vi "FP_Tracker_v.2.2+.vi"() -> ()   [LabVIEW 2018]
uses:
  SubVi's/Controls/CTL_IO_status_indicator.ctl
  SubVi's/Controls/CTL_Zones_control_and_indicator.ctl
  SubVi's/Controls/CTL_All_References.ctl
  SubVi's/Controls/CTL_Controls_References.ctl
  SubVi's/Controls/CTL_Indicators_References.ctl
  SubVi's/Controls/CTL_Panes_and_VIs_References.ctl
  SubVi's/Controls/CTL_Cage_radial_segmentation.ctl
  SubVi's/Controls/CTL_Image_Geometrical_and_scaling_parameters.ctl
  SubVi's/Controls/CTL_Control_States.ctl
  SubVi's/Controls/CTL_States_cluster.ctl
  <vilib>/Platform/TimedLoop/XDataNode/timing_clust.ctl
  <vilib>/Platform/TimedLoop/XDataNode/nitl_modes.ctl
  <vilib>/Platform/TimedLoop/XDataNode/wakeup.ctl
  <vilib>/Utility/error.llb/DialogType.ctl
  SubVi's/Controls/CTL_Acquisition_speed_selector.ctl
  <vilib>/Instr/_visa.llb/VISA Flush IO Buffer Mask.ctl
  <extravilib>/ChannelInstances/Lossy Stream-c(dbl,dbl,sgl,dbl,dbl,dbl,sgl,dbl)/Read With Abort.vi
  <extravilib>/ChannelInstances/Lossy Stream-c(dbl,dbl,sgl,dbl,dbl,dbl,sgl,dbl)/Write With Abort.vi
  <extravilib>/ChannelInstances/Lossy Stream-c(dbl,dbl,sgl,dbl,dbl,dbl,sgl,dbl)/EndpointRead.vi
  <extravilib>/ChannelInstances/Lossy Stream-c(dbl,dbl,sgl,dbl,dbl,dbl,sgl,dbl)/Endpoint.vi
  <extravilib>/ChannelInstances/Lossy Stream-c(dbl,dbl,sgl,dbl,dbl,dbl,sgl,dbl)/Instantiate.vi
  SubVi's/SW_Globals_2.2+.vi
  <vilib>/Platform/TimedLoop/scheduler/LVUserAPI/_suppVIs/Create_1kHz_TSource.vi
  <extravilib>/ChannelInstances/Lossy Stream-c(dbl,dbl,sgl,dbl,dbl,dbl,sgl,dbl)/)Channel.vi
  <resource>/ChannelSupport/_ChannelSupport/WaitIfNeeded.vi
  <vilib>/nisyscfg/Close (Resources).vi
  <vilib>/nisyscfg/Close (System).vi
  <vilib>/platform/TimedLoop/XDataNode/XDataNode.xnode
  <vilib>/Platform/TimedLoop/XDataNode/XDNodeRunTimeDep.lvlib
  <extravilib>/ChannelInstances/Lossy Stream-c(dbl,dbl,sgl,dbl,dbl,dbl,sgl,dbl).lvlib
  <vilib>/nisyscfg/nisyscfg.lvlib
  <resource>/objmgr/nisysapi.rc
  <resource>/objmgr/nicontrollersysapi.rc
  <vilib>/Utility/config.llb/NI_LVConfig.lvlib
panel:
  out "CPU load":sgl(slide) scale=0.0..100.0
  in  "ROIs list":i32(listbox)
  out "ROIs":T1
  out "Rainbow track (l.v.o.)":bool=TRUE
  out "Colors array (l.v.o.)":u32[](array[colorbox])
  out "UI update period (l.v.o.)":i64=53
  out "Trace length, samples (l.v.o)":u16(slide)=20 scale=0.0..2000.0
  out "Bright mouse lineout (l.v.o.)":bool
  out "Img geom and scaling (l.v.o.)":T2
  out "SG coeff. 0th order (l.v.o.)":dbl[](array[numeric])
  out "Ports IO config (l.v.o.)":bool[](array[boolean])
  out "SB size (l.v.o.)":u8
  out "VISA resource name":refnum<visa-resource-name>
  out "Cage size":string="Large" caption="Cage diameter"
  in  "Set/Rec and Analyse Tab":enum32{"Settings", "Recording and Analysis"}(tab)
  in  "Set IO config":bool
  in  "Save settings":bool
  in  "Reset zones":bool
  out "Ready":bool=TRUE
  in  "Check HW connection":bool
  in  "Reset stimuli":bool
  in  "Cage radial segmentation":T3={"CENTER"={"Radius, mm CENTER"=30}, "MIDFIELD"={"Radius, mm MIDFIELD"=75, "N segments MIDFIELD"=2, "Starting angle MIDFIELD"=0}, "BORDER"={"N segments BORDER"=4, "Starting angle BORDER"=0}} caption="Radial segmentation" {"BORDER"."N segments BORDER" min=1 max=12; "MIDFIELD"."N segments MIDFIELD" max=8; "CENTER"."Radius, mm CENTER" min=5 step=1}
  in  "Stimulus presets (RZ)":T4(array[cluster]) {"TTL out" items=["1"=1, "2"=2, "1 + 2"=3]; "Stimulus, s" min=0 max=10000 step=0.1; "Time, s" min=0 max=10000 step=0.1; "Event type" items=["Time spent in zone", "Future options"]}
  in  "Rainbow track":bool caption="Rainbow"
  in  "Show magnets":bool=TRUE caption="Magnets"
  in  "Playback speed":u16(ring)=3 caption="Speed" items=["25"=75, "10"=30, "6"=18, "4"=12, "2"=6, "1"=3, "2/3"=2, "1/3"=1]
  in  "Show heatmap":bool caption="Heat map"
  in  "Show full track":bool caption="Full track"
  in  "Show zones":bool=TRUE caption="Zones"
  in  "Trace, s":u16(slide)=5 max=30 step=1 scale=0.0..30.0
  out "Mouse speed, mm/s":dbl=0.28949046360238656 caption="Mouse speed" format="%05.1f"
  in  "Multiplyer of chart RX":u8(slide)=1 min=1 max=10 step=1 scale=1.0..6.0
  out "Running, perc. of time":dbl=0.28949046360238656 caption="Run, %" format="%05.2f"
  out "Mouse speed":waveform(dbl)(graph)={"t0"=timestamp(3610093053.229 s since 1904-01-01), "dt"=1.0, "Y"=[0.28949046360238656]}
  out "Histograms":dbl[](graph) caption="Zone preference (normalized)"
  in  "Reset barplot":bool
  out "Timing Source":string
  in  "Panes references":T5
  in  "Indicators references":T6
  in  "Controls references":T7
  in  "All references":T8
  in  "Experiment Diagram":T9(plugin-control)=refnum
  out "HW info":string
  out "Port":string="Large"
  in  "Timeline":dbl(slide) min=0.0 step=1.0 scale=0.0..3599.0 scale format="%<%H:%M:%S>t"
  in  "Play/Pause":bool
  in  "Open File":bool
  out "Record timestamp":dbl format="%<%H:%M:%S%3u>t"
  out "Current Time":timestamp=timestamp(3610093053.229 s since 1904-01-01) format="%<%H:%M:%S %d.%m.%Y>T"
  out "Current zone":T10={"01"=TRUE, "02"=TRUE, "03"=TRUE, "04"=TRUE, "05"=TRUE, "06"=TRUE, "07"=TRUE, "08"=TRUE, "09"=TRUE, "10"=TRUE, "11"=TRUE, "12"=TRUE, "13"=TRUE}
  in  "Record/Stop":bool
  in  "By Zone stim. setup":T11=enum."Zone 13"
  out "IO status indicator":T12
  in  "error in (no error)":errorcluster
  out "error out":errorcluster={"status"=TRUE, "code"=1, "source"="Dequeue Element in NI_LVConfig.lvlib:Read Value Without Comment.vi->NI_LVConfig.lvlib:Read Key (I32).vi->SW_Load_settings_to_main_tab.vi"}
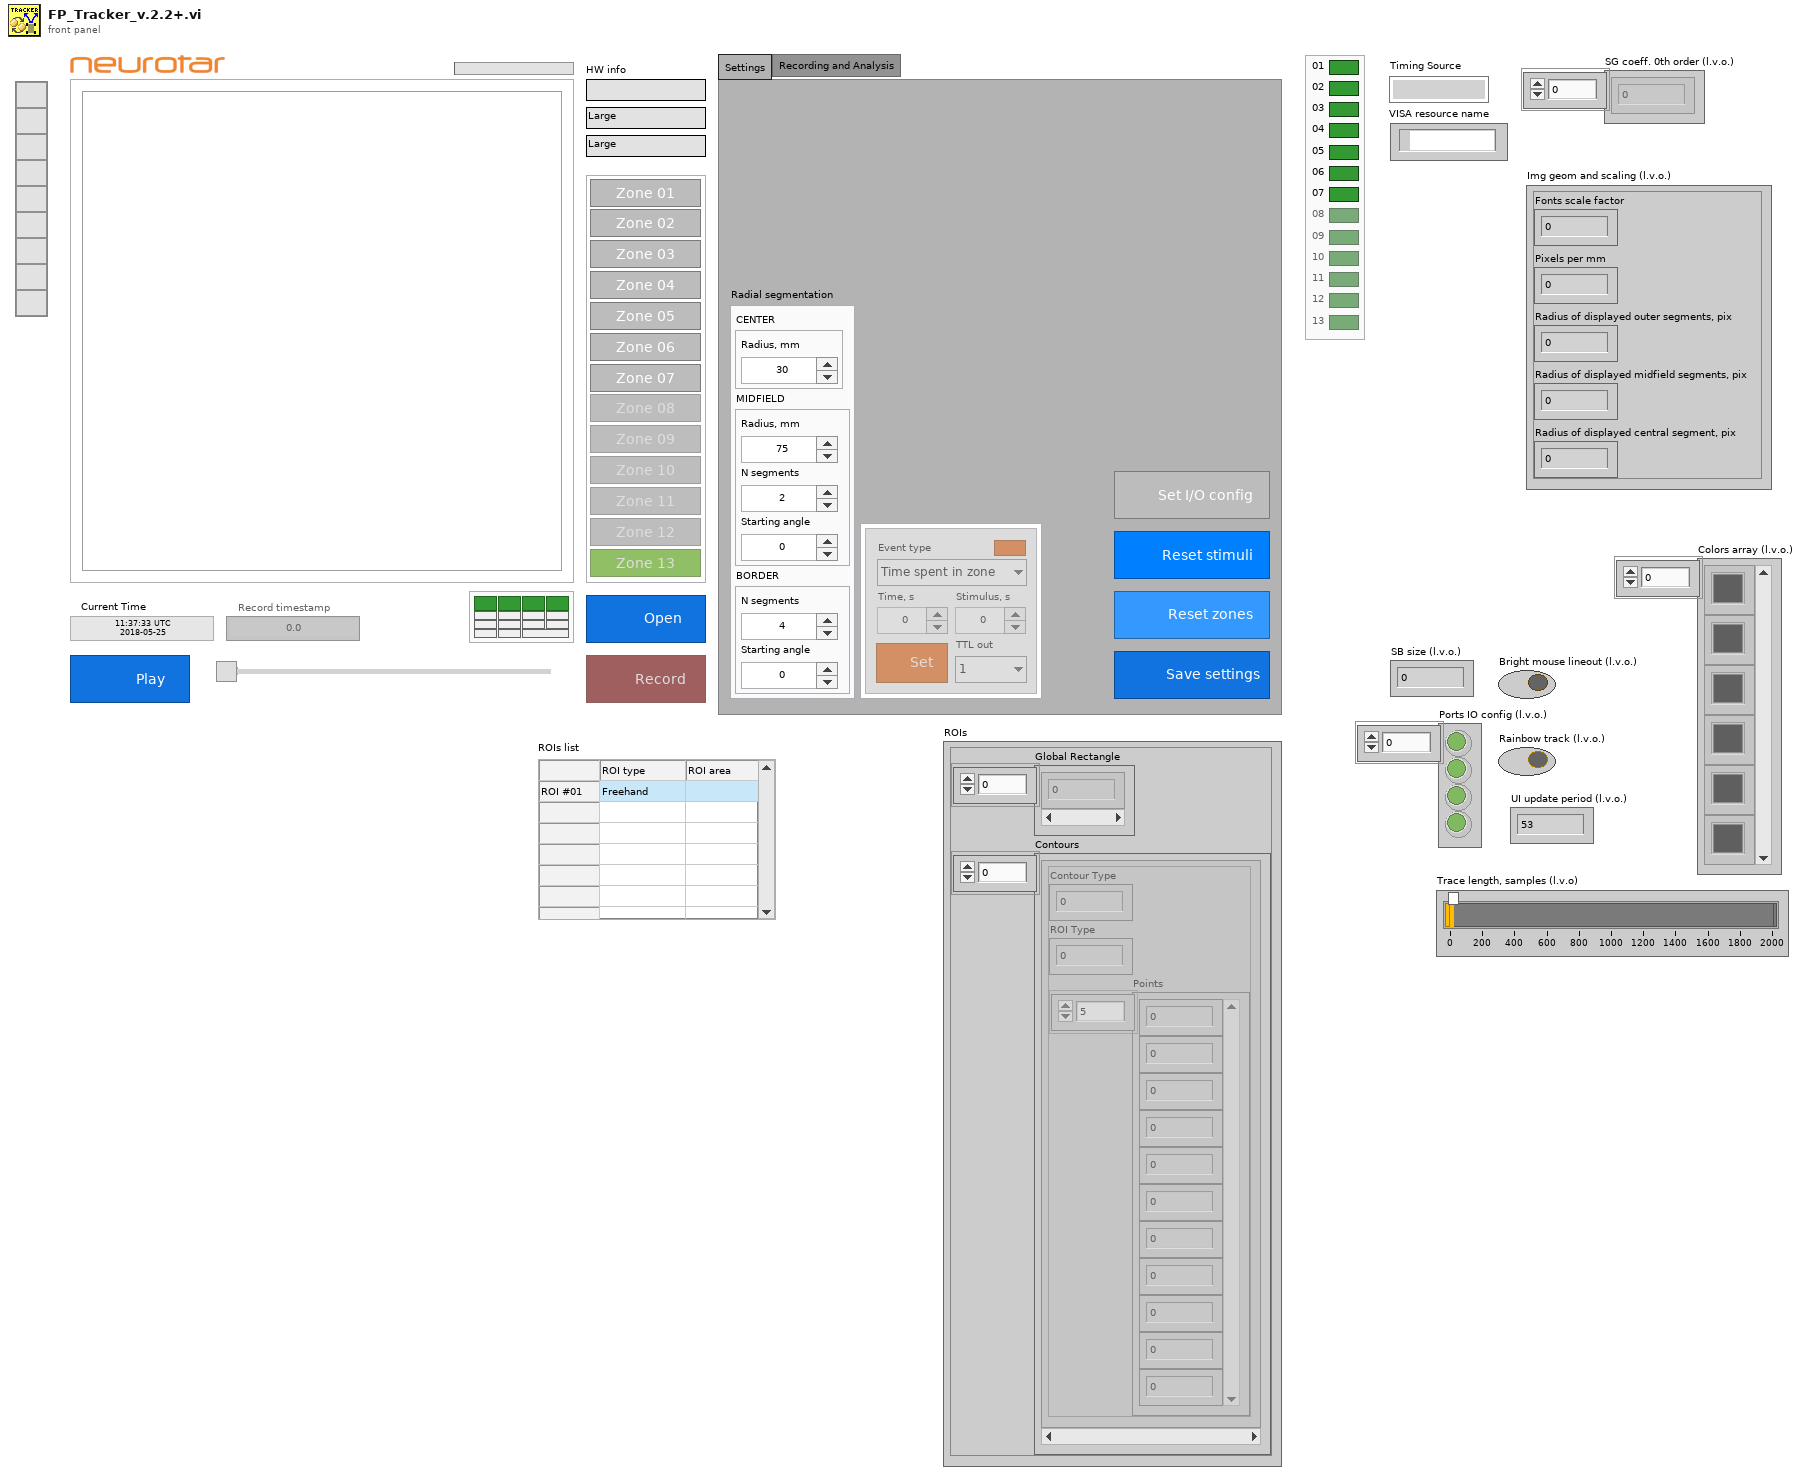
[diagram p1: front panel]
types:
  T1 = cluster{"Global Rectangle":i32[], "Contours":cluster{"Contour Type":u32, "ROI Type":u32, "Points":i32[]}[]}
  T2 = typedef "CTL_Image_Geometrical_and_scaling_parameters.ctl" = cluster{"Fonts scale factor":dbl, "Pixels per mm":dbl, "Radius of displayed outer segments, pix":dbl, "Radius of displayed midfield segments, pix":dbl, "Radius of displayed central segment, pix":dbl}
  T3 = typedef "CTL_Cage_radial_segmentation.ctl" = cluster{"CENTER":cluster{"Radius, mm CENTER":u16}, "MIDFIELD":cluster{"Radius, mm MIDFIELD":u16, "N segments MIDFIELD":u8, "Starting angle MIDFIELD":i16}, "BORDER":cluster{"N segments BORDER":u8, "Starting angle BORDER":i16}}
  T4 = cluster{"Event type":u16, "Time, s":sgl, "Stimulus, s":sgl, "Set/Clear":bool, "TTL out":u16, "Stim. has been set":bool}[]
  T5 = typedef "CTL_Panes_and_VIs_References.ctl" = cluster{"Pane":refnum<vi>, "This VI":refnum<vi>, "Menu":refnum<k9>}
  T6 = typedef "CTL_Indicators_References.ctl" = cluster{"HW info":refnum<vi>, "Port":refnum<vi>, "Ready":refnum<vi>, "IO status indicator":refnum<vi>, "Current Time":refnum<vi>, "Record timestamp":refnum<vi>, "Mouse speed":refnum<vi>, "Mouse speed, mm/s":refnum<vi>, "Running, perc. of time":refnum<vi>, "Histograms":refnum<vi>, "Cage size":refnum<vi>}
  T7 = typedef "CTL_Controls_References.ctl" = cluster{"Check HW connection":refnum<vi>, "Start Tracking button":refnum<vi>, "Reset zones":refnum<vi>, "Reset stimuli":refnum<vi>, "Record/Stop":refnum<vi>, "Reset barplot":refnum<vi>, "Multiplyer of chart RX":refnum<vi>, "Show zones":refnum<vi>, "Show magnets":refnum<vi>, "Show heatmap":refnum<vi>, "Show full track":refnum<vi>, "Open File":refnum<vi>, "Play/Pause":refnum<vi>, "Trace, s":refnum<vi>, "Playback speed":refnum<vi>, "Timeline":refnum<vi>, "By Zone stim. setup":refnum<vi>, "Set, Rec and Analyse Tab":refnum<vi>, "Cage radial segmentation":refnum<vi>, "Set IO config":refnum<vi>, "Rainbow track":refnum<vi>}
  T8 = typedef "CTL_All_References.ctl" = cluster{"Controls references":T7, "Indicators references":T6, "Service references":T5}
  T9 = typedef "IMAQ Image.ctl" = refnum<image>
  T10 = cluster{"01":bool, "02":bool, "03":bool, "04":bool, "05":bool, "06":bool, "07":bool, "08":bool, "09":bool, "10":bool, "11":bool, "12":bool, "13":bool}
  T11 = typedef "CTL_Zones_control_and_indicator.ctl" = enum32{"No Selection", "Zone 01", "Zone 02", "Zone 03", "Zone 04", "Zone 05", "Zone 06", "Zone 07", "Zone 08", "Zone 09", "Zone 10", "Zone 11", "Zone 12", "Zone 13"}
  T12 = typedef "CTL_IO_status_indicator.ctl" = cluster{"IO1":bool, "IO2":bool, "IO3":bool, "IO4":bool, "St1":bool, "St2":bool, "St3":bool, "St4":bool, "Z1":bool, "Z2":bool, "Z3":bool, "Z4":bool, "Syn1":bool, "Syn2":bool, "RS-232 ext. activated":bool}
  T13 = cluster{"HW info":refnum<vi>, "Port":refnum<vi>, "Ready":refnum<vi>, "IO status indicator":refnum<vi>, "Current Time":refnum<vi>, "Record timestamp":refnum<vi>, "Mouse speed":refnum<vi>, "Mouse speed, mm/s":refnum<vi>, "Running, perc. of time":refnum<vi>, "Histograms":refnum<vi>, "Cage size":refnum<vi>}
  T14 = cluster{"Pane":refnum<vi>, "This VI":refnum<vi>, "menu reference":refnum<k9>}
  T15 = cluster{"Check HW connection":refnum<vi>, "Save settings":refnum<vi>, "Reset zones":refnum<vi>, "Reset stimuli":refnum<vi>, "Record/Stop":refnum<vi>, "Reset barplot":refnum<vi>, "Multiplyer of chart RX":refnum<vi>, "Show zones":refnum<vi>, "Show magnets":refnum<vi>, "Show heatmap":refnum<vi>, "Show full track":refnum<vi>, "Open File":refnum<vi>, "Play/Pause":refnum<vi>, "Trace, s":refnum<vi>, "Playback speed":refnum<vi>, "Timeline":refnum<vi>, "By Zone stim. setup":refnum<vi>, "Set/Rec and Analyse Tab":refnum<vi>, "Cage radial segmentation":refnum<vi>, "Set IO config":refnum<vi>, "Rainbow track":refnum<vi>}
  T16 = typedef "CTL_States_cluster.ctl" = cluster{"Acq. is ON":bool, "Playing loaded":bool, "Recording now":bool, "Has been recorded":bool, "Data saved":bool, "Data loaded":bool, "Stop and Exit":bool}
  T17 = typedef "CTL_Control_States.ctl" = enum16{"SW Init", "HW Init", "Close App", "Update port info (Init OK)", "Unlock UI (init OK)", "Save HW Settings", "Re-check HW (init failed)", "Configure port(s)", "Zones layout update", "Set I/O config", "Reset stimulus", "Reset zones", "Play Start", "Play Stop", "Upd. trace length", "Cage and recording settings", "Update filter"}
  T18 = typedef "XDNodeRunTimeDep.lvlib/timing_clust.ctl" = cluster{"Expected End [f-1]":u64, "Actual End [f-1]":u64, "Finished Late? [f-1]":bool, "Expected End [i-1]":u64, "Actual End [i-1]":u64, "Finished Late? [i-1]":bool, "Expected Start [i]":u64, "Actual Start [i]":u64, "Expected Start [f]":u64, "Actual Start [f]":u64, "Source Name":string, "Structure Name":string, "Period":i64, "Deadline":i64, "Offset":i64, "Start":i64, "Priority":i32, "Timeout":i32, "Mode":T19, "Wakeup Reason":T20, "Error":errorcluster, "Source Type":string, "Secondary Source Type":string, "Global End Time":u64, "Global Start Time":u64, "Frame Duration":u64, "Iteration Duration":u64, "Assigned CPU":i32, "I/O Scan Engine Mode":u32}
  T19 = typedef "XDNodeRunTimeDep.lvlib/nitl_modes.ctl" = enum32{"No Change", "Process missed periods, maintain original phase", "Discard missed periods, maintain original phase", "Process missed periods, ignore original phase", "Discard missed periods, ignore original phase"}
  T20 = typedef "XDNodeRunTimeDep.lvlib/wakeup.ctl" = enum32{"Normal", "Aborted", "Asynchronous wakeup", "Timing source error", "Timed loop error", "Timeout"}
  T21 = cluster{"Contour Type":u32, "ROI Type":u32, "Points":i32[]}[]
  T22 = typedef "CTL_Settings_cluster.ctl" = cluster{"Defaults":cluster{"Default User":dbl, "VISA Resource Name ":string}, "Recording and saving":cluster{"Researcher name":string, "Name prefix":string, "Data filtering":T23, "Stop at":dbl, "\"Stop at\" enabled":bool, "Default save folder path":path}, "Geometry":T24, "IO parameters":T25, "Stimulus presets array":T26[], "Settings loaded OK":bool}
  T23 = typedef "CTL_Filter_selector.ctl" = cluster{"Filter type":enum16{"None", "Savitzky-Golay"}, "Length":i32, "Order":i32}
  T24 = typedef "CTL_Segmented_plot_parameters.ctl" = cluster{"Cage diameter, mm":u16, "Starting angle MIDFIELD":i16, "Starting angle BORDER":i16, "Radius, mm CENTER":u16, "Radius, mm MIDFIELD":u16, "N segments MIDFIELD":u8, "N segments BORDER":u8, "R-gap, mm":sgl, "Bridge swap":bool, "Bridge H. offset":sgl, "Bridge V. offset":sgl, "Twisted neck":bool, "Alt. magn. orientation":bool}
  T25 = typedef "CTL_IO_params_cluster.ctl" = cluster{"IO general config.":u16, "IO 1 configuration":u16, "IO 2 configuration":u16, "IO 3 configuration":u16, "IO 4 configuration":u16, "Activate ext. RS-232":u16, "IO inversion config.":u16, "Sync capability":u8}
  T26 = typedef "CTL_Single_stimulus_setting.ctl" = cluster{"Event type":u16, "Dur., s":sgl, "Stim., s":sgl, "TTL out N":u16, "Set/Clear":bool, "Stim. has been set":bool}
  T27 = cluster{"Radius, mm MIDFIELD":u16, "N segments MIDFIELD":u8, "Starting angle MIDFIELD":i16}
  T28 = cluster{"N segments BORDER":u8, "Starting angle BORDER":i16}
  T29 = cluster{"Numeric Control":u32, "Numeric Control":u32}[]
  T30 = typedef "CTL_Acquisition_speed_selector.ctl" = enum16{"Max", "High stability", "Eco"}
  T31 = enum32{"Page Enabled", "Page Disabled", "Page Disabled & Grayed"}
  T32 = enum8{"Enabled", "Disabled", "Disabled and Grayed Out"}
  T33 = typedef "DialogType.ctl" = u16
  T34 = enum32{"invalid app kind", "Development System", "Run Time System", "Student Edition", "Embedded LabVIEW", "Evaluation", "Custom"}
  T35 = typedef "CTL_Paths_cluster.ctl" = cluster{"Temporary file output path":path, "Density map array output path":path, "Recording settings output path":path, "Density map picture output path":path, "Layout picture output path":path, "Path to the settings file":path, "Path to TDMS file":path, "TDMS file reference":refnum<k34>, "Default save folder path":path}
  T36 = cluster{"Default User":dbl, "VISA Resource Name ":string}
  T37 = typedef "NI_LVConfig.lvlib/Config Data RefNum.ctl" = refnum<k1>
  T38 = typedef "VISA Flush IO Buffer Mask.ctl" = u16
  T39 = cluster{"ms since ON":u32, "delta time":u32, "X1":sgl, "Y1":sgl, "X2":sgl, "Y2":sgl, "TTL inputs":u8, "TTL outputs":u8, "Frame timestamp":timestamp, "Frame OK":bool}
  T40 = cluster{"ms since ON":u32, "delta time":u32, "X1":sgl, "Y1":sgl, "X2":sgl, "Y2":sgl, "TTL in 1":i16, "TTL in 2":i16, "Frame timestamp":timestamp, "Frame OK":bool}
  T41 = cluster{"R from center":dbl, "sin(a)":dbl, "Mouse Xc":dbl, "Mouse Yc":dbl, "X1-X2":dbl, "Y1-Y2":dbl, "Cage Xc":dbl, "Cage Yc":dbl}
  T42 = cluster{"R from center":dbl, "phi (mouse angular position in the cage)":dbl, "alpha (mouse rot. angle)":sgl, "X":dbl, "Y":dbl, "theta (from center towards mouse)":dbl, "beta (cage rot. against mouse)":sgl, "w (mouse angle to wall)":dbl}
  T43 = typedef "Lossy Stream-c(dbl,dbl,sgl,dbl,dbl,dbl,sgl,dbl).lvlib/)Channel.ctl" = refnum<queue>
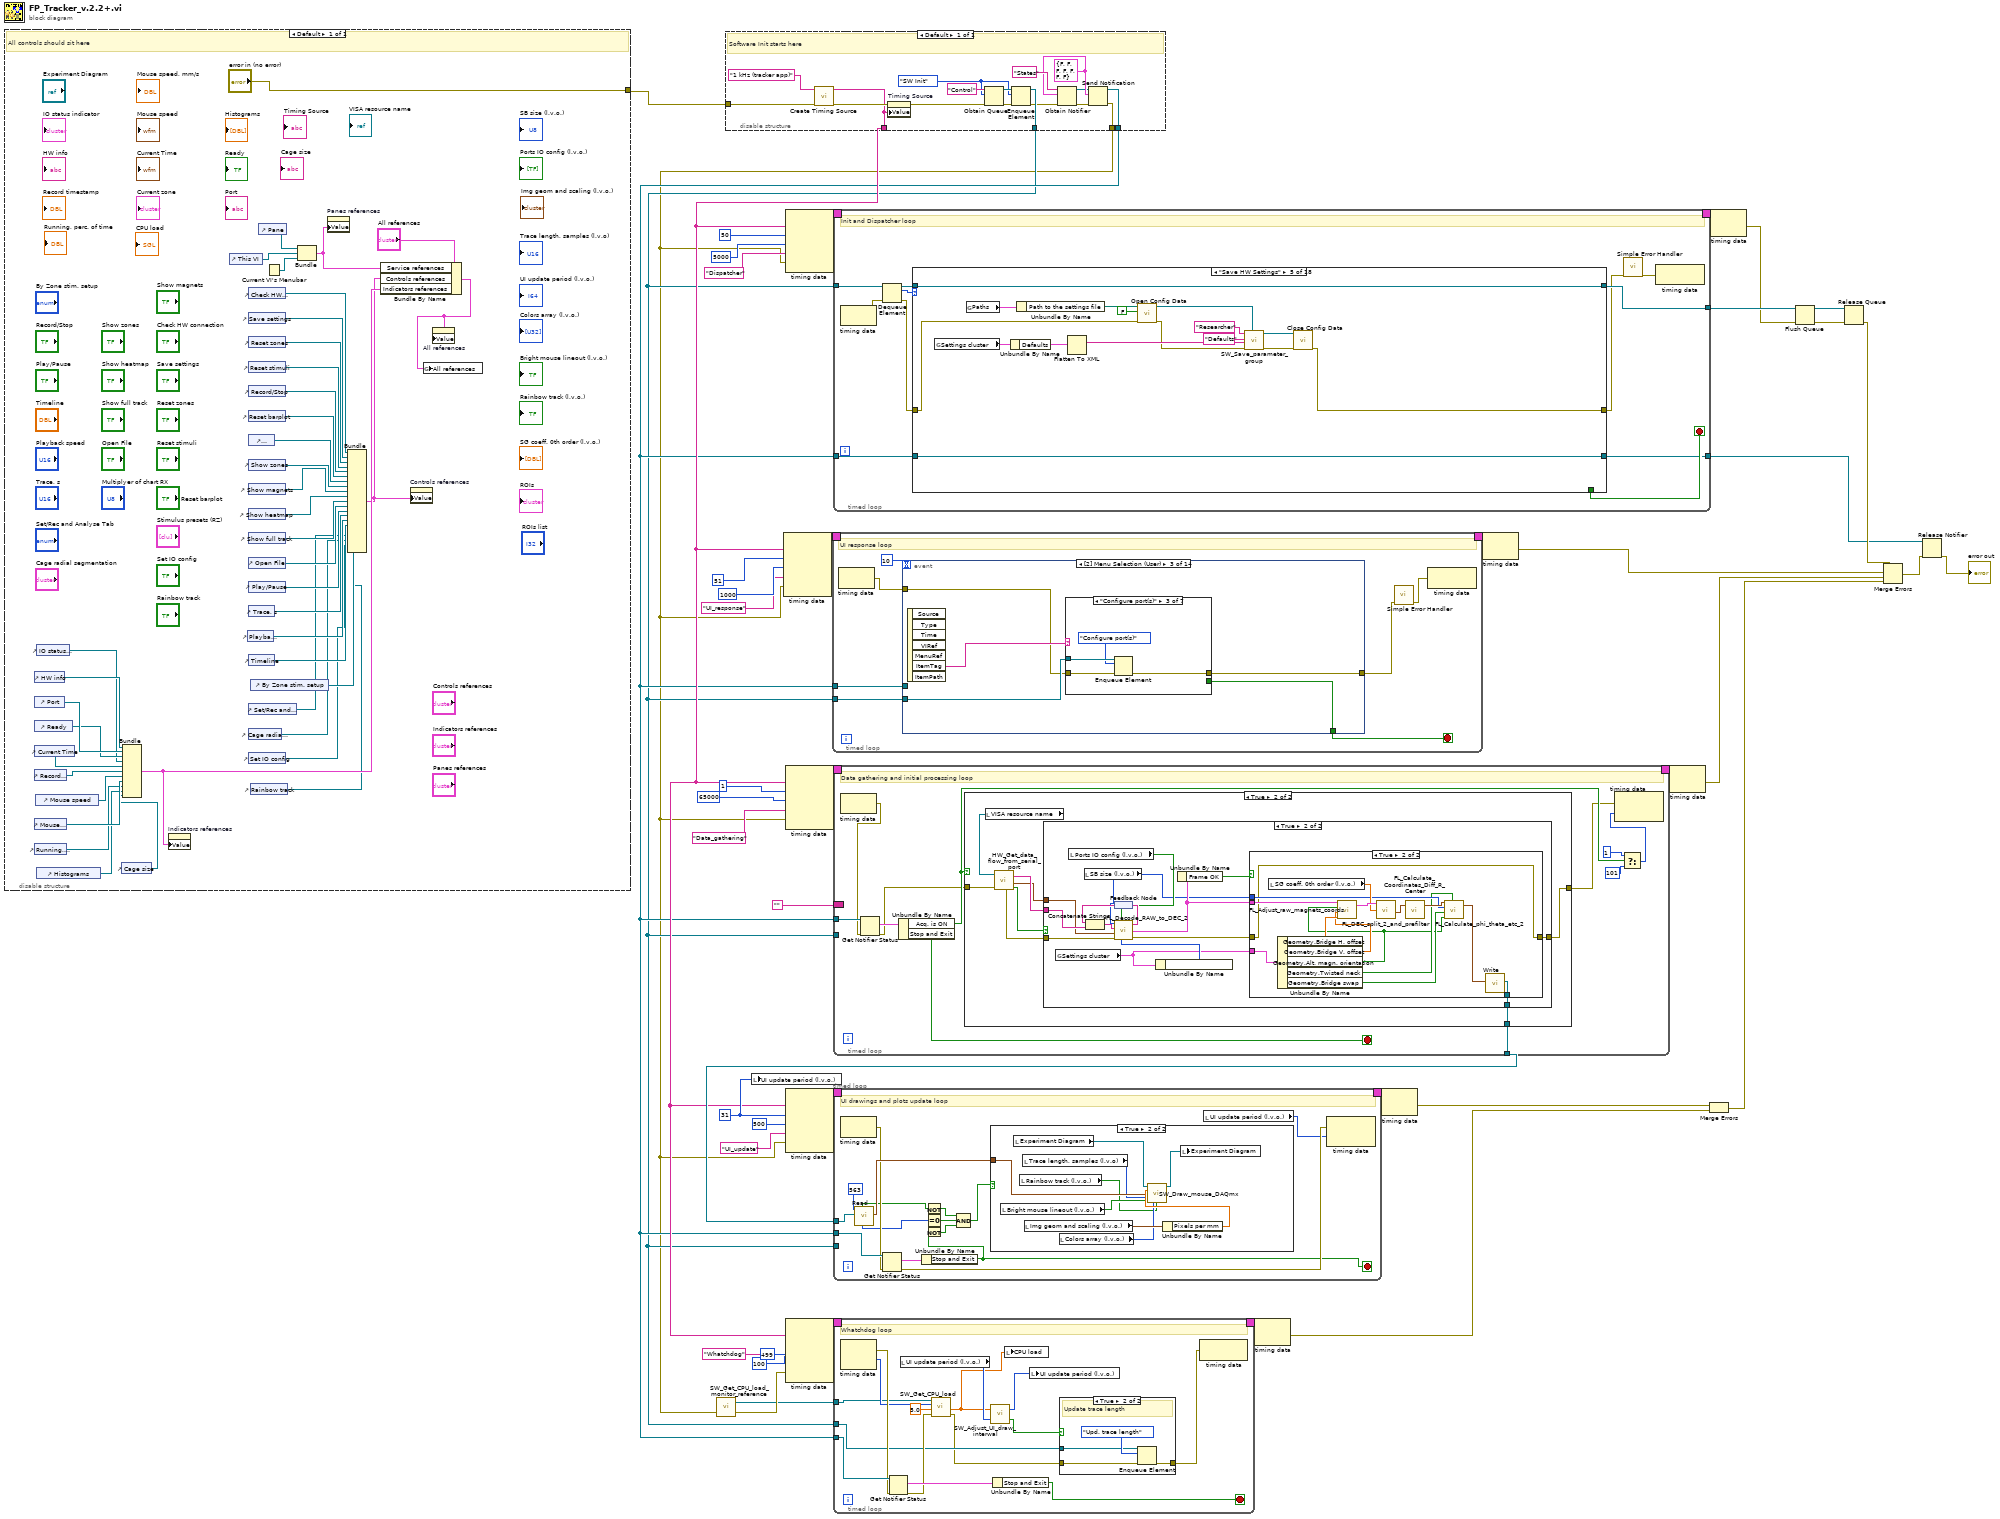
[diagram p0: block diagram]
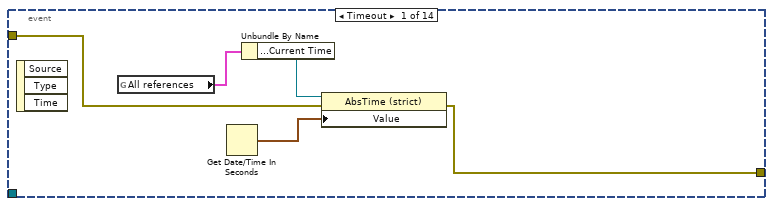
[diagram p7: hidden frame]
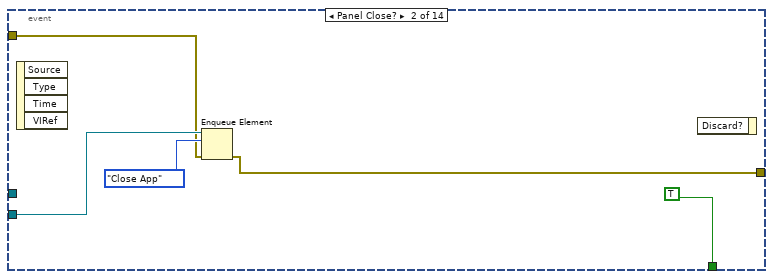
[diagram p8: hidden frame]
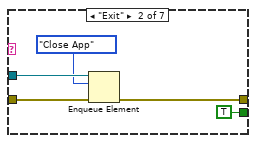
[diagram p10: hidden frame]
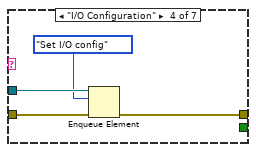
[diagram p11: hidden frame]
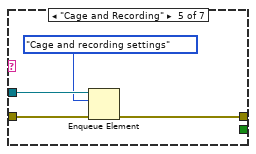
[diagram p12: hidden frame]
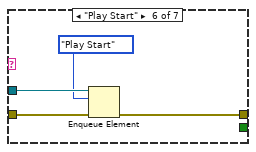
[diagram p13: hidden frame]
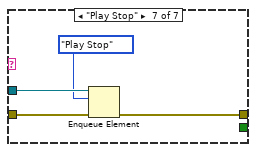
[diagram p14: hidden frame]
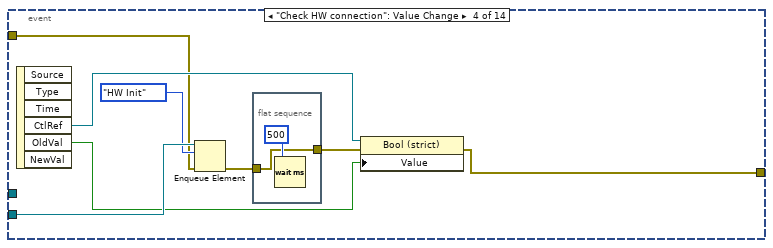
[diagram p15: hidden frame]
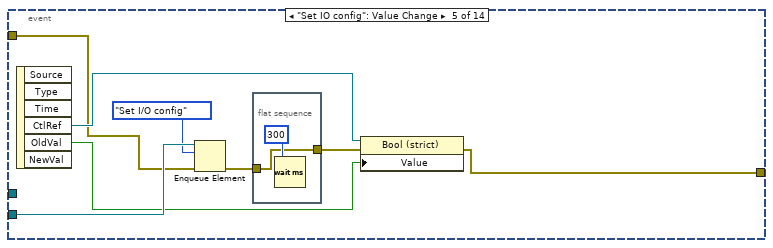
[diagram p16: hidden frame]
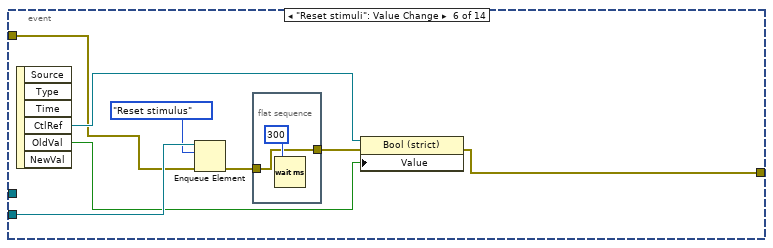
[diagram p17: hidden frame]
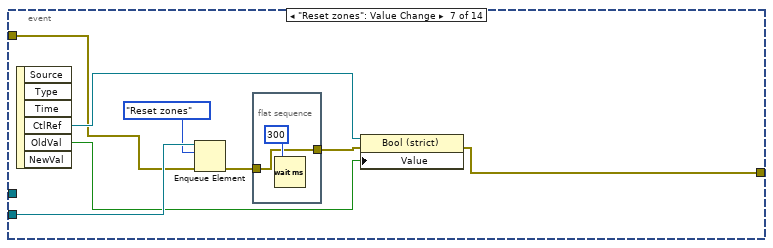
[diagram p18: hidden frame]
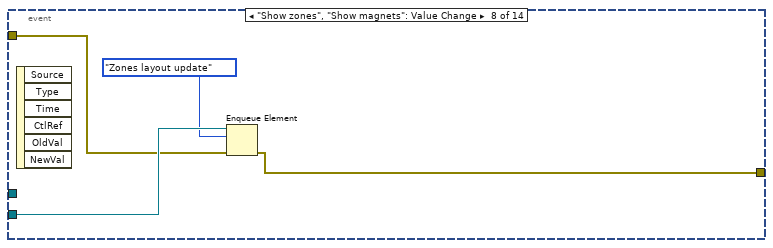
[diagram p19: hidden frame]
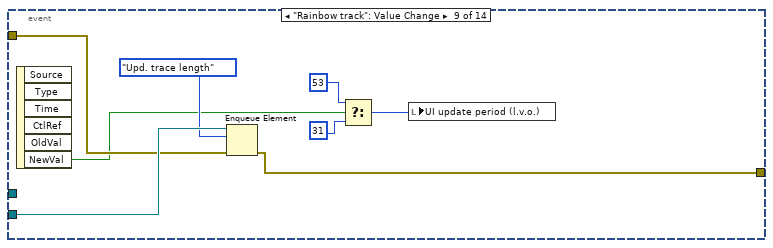
[diagram p20: hidden frame]
diagram:
  w23 = i64 31 ("Period")
  n1 = disable-structure shown="Default" {
    disable-tunnel: ["error in (no error)"] -> w29
    frame Enabled {
      # "All controls should sit here"
      n2 = control-ref of="Record timestamp"() -> (w67:refnum<vi>)
      n3 = control-ref of="Mouse speed, mm/s"() -> (w65:refnum<vi>)
      n4 = control-ref of="Running, perc. of time"() -> (w64:refnum<vi>)
      n5 = control-ref of="HW info"() -> (w71:refnum<vi>)
      n6 = control-ref of="Port"() -> (w70:refnum<vi>)
      n7 = control-ref of="Ready"() -> (w69:refnum<vi>)
      n8 = control-ref of="Current Time"() -> (w68:refnum<vi>)
      n9 = control-ref of="Mouse speed"() -> (w66:refnum<vi>)
      n10 = control-ref of="IO status indicator"() -> (w59:refnum<vi>)
      n11 = control-ref of="Histograms"() -> (w63:refnum<vi>)
      n12 = control-ref of="Cage size"() -> (w50:refnum<vi>)
      n13 = Bundle("HW info"=w71, "Port"=w70, "Ready"=w69, "IO status indicator"=w59, "Current Time"=w68, "Record timestamp"=w67, "Mouse speed"=w66, "Mouse speed, mm/s"=w65, "Running, perc. of time"=w64, "Histograms"=w63, "Cage size"=w50) -> (w56:T13)  [unwired: 1 in]
      n14 = property on="Indicators references" class="Clust (strict)"("Value"=w56) -> ()  [unwired: 2 in, 2 out]
      n15 = control-ref of="This VI"() -> (w61:refnum<vi>)
      n16 = control-ref of="Playback speed"() -> (w74:refnum<vi>)
      n17 = control-ref of="Check HW connection"() -> (w87:refnum<vi>)
      n18 = control-ref of="Save settings"() -> (w86:refnum<vi>)
      n19 = control-ref of="Reset zones"() -> (w85:refnum<vi>)
      n20 = control-ref of="Reset stimuli"() -> (w84:refnum<vi>)
      n21 = control-ref of="Record/Stop"() -> (w83:refnum<vi>)
      n22 = control-ref of="Reset barplot"() -> (w82:refnum<vi>)
      n23 = control-ref of="Multiplyer of chart RX"() -> (w81:refnum<vi>)
      n24 = control-ref of="Show zones"() -> (w80:refnum<vi>)
      n25 = control-ref of="Show magnets"() -> (w60:refnum<vi>)
      n26 = control-ref of="Show heatmap"() -> (w79:refnum<vi>)
      n27 = control-ref of="Show full track"() -> (w78:refnum<vi>)
      n28 = control-ref of="Open File"() -> (w77:refnum<vi>)
      n29 = control-ref of="Play/Pause"() -> (w76:refnum<vi>)
      n30 = control-ref of="Trace, s"() -> (w75:refnum<vi>)
      n31 = control-ref of="Timeline"() -> (w73:refnum<vi>)
      n32 = control-ref of="Set/Rec and Analyse Tab"() -> (w54:refnum<vi>)
      n33 = control-ref of="Cage radial segmentation"() -> (w53:refnum<vi>)
      n34 = control-ref of="Set IO config"() -> (w52:refnum<vi>)
      n35 = control-ref of="By Zone stim. setup"() -> (w72:refnum<vi>)
      n36 = control-ref of="Rainbow track"() -> (w48:refnum<vi>)
      n37 = control-ref of="Pane"() -> (w62:refnum<vi>)
      n38 = Current VI's Menubar() -> (w49:refnum<k9>)
      n39 = Bundle("Pane"=w62, "This VI"=w61, "menu reference"=w49) -> (w57:T14)  [unwired: 1 in]
      n40 = property on="Panes references" class="Clust (strict)"("Value"=w57) -> ()  [unwired: 2 in, 2 out]
      n41 = Bundle("Check HW connection"=w87, "Save settings"=w86, "Reset zones"=w85, "Reset stimuli"=w84, "Record/Stop"=w83, "Reset barplot"=w82, "Multiplyer of chart RX"=w81, "Show zones"=w80, "Show magnets"=w60, "Show heatmap"=w79, "Show full track"=w78, "Open File"=w77, "Play/Pause"=w76, "Trace, s"=w75, "Playback speed"=w74, "Timeline"=w73, "By Zone stim. setup"=w72, "Set/Rec and Analyse Tab"=w54, "Cage radial segmentation"=w53, "Set IO config"=w52, "Rainbow track"=w48) -> (w51:T15)  [unwired: 1 in]
      n42 = Bundle By Name(cluster="All references", "Service references"=w57, "Controls references"=w51, "Indicators references"=w56) -> (w55:T8)
      n43 = property on="Controls references" class="Clust (strict)"("Value"=w51) -> ()  [unwired: 2 in, 2 out]
      n44 = global write "SW_Globals_2.2+.vi" "All references"(w55) -> ()
      n45 = property on="All references" class="Clust (strict)"("Value"=w55) -> ()  [unwired: 2 in, 2 out]
    }
  }
  n46 = disable-structure shown="Default" {
    disable-tunnel: w29 -> [w98]
    disable-tunnel: [w97] -> w6
    disable-tunnel: [w96] -> w11
    disable-tunnel: [w90] -> w7
    disable-tunnel: [w89] -> w3
    frame Enabled {
      w92 = T16 {"Acq. is ON"=FALSE, "Playing loaded"=FALSE, "Recording now"=FALSE, "Has been recorded"=FALSE, "Data saved"=FALSE, "Data loaded"=FALSE, "Stop and Exit"=FALSE} ("States cluster")
      w99 = CTL_Control_States."SW Init"
      # "Software Init starts here"
      n47 = call-poly <vilib>:"Create Timing Source.vi"("error in (no error)"=w98, "name (in)"="1 kHz (tracker app)") -> ("error out"=w105:errorcluster, "name (out)"=w96:string)  [unwired: 8 in]
      n48 = property on="Timing Source" class="Str"(error in=w105, "Value"=w96) -> (error out=w103:errorcluster)  [unwired: 1 in, 1 out]
      n49 = Obtain Queue(name (unnamed)="Control", element data type=w99, error in (no error)=w103) -> (queue out=w100:refnum<queue>, error out=w101:errorcluster)  [unwired: 2 in, 1 out]
      n50 = Enqueue Element(queue=w100, element=w99, error in (no error)=w101) -> (queue out=w97:refnum<queue>, error out=w95:errorcluster)  [unwired: 1 in, 1 out]
      n51 = Obtain Notifier(name (unnamed)="States", notification data type=w92, error in (no error)=w95) -> (notifier out=w91:refnum<notifier>, error out=w93:errorcluster)  [unwired: 1 in, 1 out]
      n52 = Send Notification(notification=w92, notifier=w91, error in (no error)=w93) -> (notifier out=w90:refnum<notifier>, error out=w89:errorcluster)
    }
  }
  n53 = call "SW_Get_CPU_load_monitor_reference.vi"("error in (no error)"=w3) -> ("error out"=w2:errorcluster, "CPU monitor .NET reference"=w1:refnum<k24>)  [unwired: 1 in]
  n54 = local write "UI update period (l.v.o.)"(w23) -> ()
  n55 = node-c288(w11, i64 51 ("Period"), 1000 ("Priority"), "UI_response" ("Structure Name"), w3) -> (w40:T18)
  n56 = node-c288(w11, i64 50 ("Period"), 5000 ("Priority"), "Dispatcher" ("Structure Name"), w3) -> (w47:T18)
  n57 = node-c288(w11, i64 1 ("Period"), 65000 ("Priority"), "Data_gathering" ("Structure Name"), w3) -> (w35:T18)
  n58 = node-c288(w11, w23, 500 ("Priority"), "UI_update" ("Structure Name"), w3) -> (w28:T18)
  n59 = node-c288(w11, i64 499 ("Period"), 100 ("Priority"), "Whatchdog" ("Structure Name"), w2) -> (w13:T18)
  n60 = timed-loop {
    timing: w40 -> [_]
    timing-out: [_] -> w39
    tunnel: w6 -> [w111]
    tunnel: w7 -> [w109]
    stop <- w112 stop-if-true
    # "UI response loop"
    n61 = node-c288() -> (w107:errorcluster)  [unwired: 1 in]
    n62 = event shown="[2] Menu Selection (User)" {
      selector: _ -> [_ _ _ _ _ _ _ _ _ _ _ _ _ _]
      dyn-events: _ -> [_ _ _ _ _ _ _ _ _ _ _ _ _ _]
      timeout: 10 -> [_ _ _ _ _ _ _ _ _ _ _ _ _ _]
      tunnel: [_ TRUE w125 _ _ _ _ _ _ _ _ _ _ _] -> w112
      tunnel: w111 -> [_ w121 w126 w161 w171 w181 w191 w197 w205 _ w234 w254 w266 w269]
      tunnel: w109 -> [_ _ _ _ _ _ _ _ _ _ _ _ _ _]
      tunnel: w107 -> [w114 w119 w124 w154 w165 w175 w185 w195 w203 w214 w231 w252 w264 w268]
      tunnel: [w113 w118 w123 w155 w164 w174 w184 w194 w202 w206 w230 w251 w263 w267] -> w106
      event Timeout {
        n63 = event-data() -> ()  [unwired: 1 in, 3 out]
        n64 = global read "SW_Globals_2.2+.vi" "All references"() -> (w116:T8)
        n65 = Get Date/Time In Seconds() -> (seconds since 1Jan1904=w117:timestamp)
        n66 = Unbundle By Name(w116) -> ("Indicators references.Current Time"=w115:refnum<vi>)
        n67 = property class="AbsTime (strict)"(reference=w115, error in=w114, "Value"=w117) -> (error out=w113:errorcluster)  [unwired: 1 out]
      }
      event Panel Close? {
        n68 = event-data() -> ()  [unwired: 1 in, 4 out]
        n69 = Enqueue Element(queue=w121, element=CTL_Control_States."Close App", error in (no error)=w119) -> (error out=w118:errorcluster)  [unwired: 1 in, 2 out]
        n70 = event-data() -> ()  [unwired: 2 in, 1 out]
      }
      event Menu Selection (User) {
        n71 = event-data() -> ("ItemTag"=w127:string)  [unwired: 1 in, 6 out]
        n72 = case shown="\"Configure port(s)\"" w127 {
          tunnel: w126 -> [_ w133 w137 w141 w145 w149 w153]
          tunnel: [_ TRUE _ _ _ _ _] -> w125
          tunnel: w124 -> [w128 w130 w135 w139 w143 w147 w151]
          tunnel: [w128 w129 w134 w138 w142 w146 w150] -> w123
          frame "", Default {
          }
          frame "Exit" {
            n73 = Enqueue Element(queue=w133, element=CTL_Control_States."Close App", error in (no error)=w130) -> (error out=w129:errorcluster)  [unwired: 1 in, 2 out]
          }
          frame "Configure port(s)" {
            n74 = Enqueue Element(queue=w137, element=CTL_Control_States."Configure port(s)", error in (no error)=w135) -> (error out=w134:errorcluster)  [unwired: 1 in, 2 out]
          }
          frame "I/O Configuration" {
            n75 = Enqueue Element(queue=w141, element=CTL_Control_States."Set I/O config", error in (no error)=w139) -> (error out=w138:errorcluster)  [unwired: 1 in, 2 out]
          }
          frame "Cage and Recording" {
            n76 = Enqueue Element(queue=w145, element=CTL_Control_States."Cage and recording settings", error in (no error)=w143) -> (error out=w142:errorcluster)  [unwired: 1 in, 2 out]
          }
          frame "Play Start" {
            n77 = Enqueue Element(queue=w149, element=CTL_Control_States."Play Start", error in (no error)=w147) -> (error out=w146:errorcluster)  [unwired: 1 in, 2 out]
          }
          frame "Play Stop" {
            n78 = Enqueue Element(queue=w153, element=CTL_Control_States."Play Stop", error in (no error)=w151) -> (error out=w150:errorcluster)  [unwired: 1 in, 2 out]
          }
        }
      }
      event "Check HW connection": Value Change {
        n79 = event-data() -> ("CtlRef"=w156:refnum<vi>, "OldVal"=w157:bool)  [unwired: 1 in, 4 out]
        n80 = Enqueue Element(queue=w161, element=CTL_Control_States."HW Init", error in (no error)=w154) -> (error out=w159:errorcluster)  [unwired: 1 in, 2 out]
        n81 = flat-sequence {
          tunnel: w159 -> [w162]
          tunnel: [w162] -> w158
          frame #0 {
            n82 = Wait (ms)(milliseconds to wait=u32 500) -> ()  [unwired: 1 out]
          }
        }
        n83 = property class="Bool (strict)"(reference=w156, error in=w158, "Value"=w157) -> (error out=w155:errorcluster)  [unwired: 1 out]
      }
      event "Set IO config": Value Change {
        n84 = event-data() -> ("CtlRef"=w166:refnum<vi>, "OldVal"=w167:bool)  [unwired: 1 in, 4 out]
        n85 = Enqueue Element(queue=w171, element=CTL_Control_States."Set I/O config", error in (no error)=w165) -> (error out=w169:errorcluster)  [unwired: 1 in, 2 out]
        n86 = flat-sequence {
          tunnel: w169 -> [w172]
          tunnel: [w172] -> w168
          frame #0 {
            n87 = Wait (ms)(milliseconds to wait=u32 300) -> ()  [unwired: 1 out]
          }
        }
        n88 = property class="Bool (strict)"(reference=w166, error in=w168, "Value"=w167) -> (error out=w164:errorcluster)  [unwired: 1 out]
      }
      event "Reset stimuli": Value Change {
        n89 = event-data() -> ("CtlRef"=w176:refnum<vi>, "OldVal"=w177:bool)  [unwired: 1 in, 4 out]
        n90 = Enqueue Element(queue=w181, element=CTL_Control_States."Reset stimulus", error in (no error)=w175) -> (error out=w179:errorcluster)  [unwired: 1 in, 2 out]
        n91 = flat-sequence {
          tunnel: w179 -> [w182]
          tunnel: [w182] -> w178
          frame #0 {
            n92 = Wait (ms)(milliseconds to wait=u32 300) -> ()  [unwired: 1 out]
          }
        }
        n93 = property class="Bool (strict)"(reference=w176, error in=w178, "Value"=w177) -> (error out=w174:errorcluster)  [unwired: 1 out]
      }
      event "Reset zones": Value Change {
        n94 = event-data() -> ("CtlRef"=w186:refnum<vi>, "OldVal"=w187:bool)  [unwired: 1 in, 4 out]
        n95 = Enqueue Element(queue=w191, element=CTL_Control_States."Reset zones", error in (no error)=w185) -> (error out=w189:errorcluster)  [unwired: 1 in, 2 out]
        n96 = flat-sequence {
          tunnel: w189 -> [w192]
          tunnel: [w192] -> w188
          frame #0 {
            n97 = Wait (ms)(milliseconds to wait=u32 300) -> ()  [unwired: 1 out]
          }
        }
        n98 = property class="Bool (strict)"(reference=w186, error in=w188, "Value"=w187) -> (error out=w184:errorcluster)  [unwired: 1 out]
      }
      event "Show zones", "Show magnets": Value Change {
        n99 = event-data() -> ()  [unwired: 1 in, 6 out]
        n100 = Enqueue Element(queue=w197, element=CTL_Control_States."Zones layout update", error in (no error)=w195) -> (error out=w194:errorcluster)  [unwired: 1 in, 2 out]
      }
      event "Rainbow track": Value Change {
        n101 = event-data() -> ("NewVal"=w201:bool)  [unwired: 1 in, 5 out]
        n102 = Enqueue Element(queue=w205, element=CTL_Control_States."Upd. trace length", error in (no error)=w203) -> (error out=w202:errorcluster)  [unwired: 1 in, 2 out]
        n103 = Select(t=i64 53 ("Period"), s=w201, f=i64 31 ("Period")) -> (s? t:f=w200:i64)
        n104 = local write "UI update period (l.v.o.)"(w200) -> ()
      }
      event "Experiment Diagram": Mouse Up {
        n105 = event-data() -> ()  [unwired: 1 in, 8 out]
        n106 = property on="Experiment Diagram" class="ImageControl"(error in=w214) -> (error out=w207:errorcluster, "ROI"=w213:T1)  [unwired: 1 in, 1 out]
        n107 = local write "ROIs"(w213) -> ()
        n108 = Unbundle By Name(w213) -> ("Contours"=w212:T21)
        n109 = for {
          tunnel: w212 -> [w222] mode=indexing
          tunnel: [w219] -> w210 mode=indexing
          tunnel: [w215] -> w211 mode=indexing
          i -> [w221]
          n110 = Unbundle By Name(w222) -> ("ROI Type"=w216:u32)
          n111 = Increment(x=w221) -> (x+1=w220:i32)
          n112 = case shown="0, Default" w216 {
            tunnel: ["Unknown" "Rect" "Rot. rect" "Polygon" "Freehand" "Oval" "Annulus"] -> w215
            frame 0, Default {
            }
            frame 3 {
            }
            frame 12 {
            }
            frame 5 {
            }
            frame 6 {
            }
            frame 4 {
            }
            frame 7 {
            }
          }
          n113 = Format Value(string ("")="ROI #" ("string"), format string="%02u", value (0)=w220) -> (output string=w219:string)
        }
        n114 = Build Array(w211) -> (w209:string[][])
        n115 = Transpose 2D Array(2D array=w209) -> (transposed array=w208:string[][])
        n116 = property on="ROIs list" class="MCListbox (strict)"(error in=w207, "ItemNames"=w208, "RowHdrs[]"=w210) -> (error out=w206:errorcluster)  [unwired: 1 in, 1 out]
      }
      event Value Change {
        n117 = event-data() -> ("CtlRef"=w246:refnum<vi>)  [unwired: 1 in, 5 out]
        n118 = global read "SW_Globals_2.2+.vi" "Settings cluster"() -> (w248:T22)
        n119 = property class="Clust (strict)"(reference=w246, error in=w231) -> (error out=w235:errorcluster, "Value"=w245:T3)  [unwired: 1 out]
        n120 = Unbundle(w245) -> ("CENTER"=w244:cluster{"Radius, mm CENTER":u16}, "MIDFIELD"=w242:T27, "BORDER"=w238:T28)
        n121 = Unbundle(w244) -> ("Radius, mm CENTER"=w243:u16)
        n122 = Unbundle(w242) -> ("Radius, mm MIDFIELD"=w241:u16, "N segments MIDFIELD"=w240:u8, "Starting angle MIDFIELD"=w239:i16)
        n123 = Unbundle(w238) -> ("N segments BORDER"=w237:u8, "Starting angle BORDER"=w236:i16)
        n124 = Bundle By Name(cluster=w248, "Geometry.Radius, mm CENTER"=w243, "Geometry.Radius, mm MIDFIELD"=w241, "Geometry.N segments MIDFIELD"=w240, "Geometry.Starting angle MIDFIELD"=w239, "Geometry.N segments BORDER"=w237, "Geometry.Starting angle BORDER"=w236) -> (w247:T22)
        n125 = global write "SW_Globals_2.2+.vi" "Settings cluster"(w247) -> ()
        n126 = flat-sequence {
          tunnel: w235 -> [w249]
          tunnel: [w249] -> w233
          frame #0 {
            n127 = Wait (ms)(milliseconds to wait=u32 100) -> ()  [unwired: 1 out]
          }
        }
        n128 = Enqueue Element(queue=w234, element=CTL_Control_States."Zones layout update", error in (no error)=w233) -> (error out=w230:errorcluster)  [unwired: 1 in, 2 out]
      }
      event "Play/Pause": Value Change {
        n129 = event-data() -> ("NewVal"=w253:bool)  [unwired: 1 in, 5 out]
        n130 = case shown="False" w253 {
          tunnel: w254 -> [w258 w262]
          tunnel: w252 -> [w256 w260]
          tunnel: [w255 w259] -> w251
          frame True {
            # "Play Start"
            n131 = Enqueue Element(queue=w258, element=CTL_Control_States."Play Start", error in (no error)=w256) -> (error out=w255:errorcluster)  [unwired: 1 in, 2 out]
          }
          frame False {
            # "Play Start"
            n132 = Enqueue Element(queue=w262, element=CTL_Control_States."Play Stop", error in (no error)=w260) -> (error out=w259:errorcluster)  [unwired: 1 in, 2 out]
          }
        }
      }
      event "Trace, s": Value Change {
        n133 = event-data() -> ()  [unwired: 1 in, 6 out]
        n134 = Enqueue Element(queue=w266, element=CTL_Control_States."Upd. trace length", error in (no error)=w264) -> (error out=w263:errorcluster)  [unwired: 1 in, 2 out]
      }
      event Value Change {
        n135 = event-data() -> ("NewVal"=w271:T11)  [unwired: 1 in, 5 out]
        n136 = To Unsigned Byte Integer(number=w271) -> (unsigned 8bit integer=w272:u8)
        n137 = Build Array(w272) -> (w270:u8[])
        n138 = flat-sequence {
          tunnel: w270 -> [w273]
          tunnel: w269 -> [w277]
          tunnel: w268 -> [w276]
          tunnel: [w275] -> w267
          frame #0 {
            n139 = global write "SW_Globals_2.2+.vi" "Regions to mark selected"(w273) -> ()
          }
          frame #1 {
            n140 = Wait (ms)(milliseconds to wait=u32 50) -> ()  [unwired: 1 out]
          }
          frame #2 {
            n141 = Enqueue Element(queue=w277, element=CTL_Control_States."Zones layout update", error in (no error)=w276) -> (error out=w275:errorcluster)  [unwired: 1 in, 2 out]
          }
        }
      }
    }
    n142 = call <vilib>:"Simple Error Handler.vi"("error in (no error)"=w106) -> ("error out"=w108:errorcluster)  [unwired: 4 in, 4 out]
    n143 = node-c288(w108) -> ()  [unwired: 1 out]
  }
  n144 = timed-loop {
    timing: w47 -> [_]
    timing-out: [_] -> w46
    tunnel: w6 -> [w294]
    tunnel: [w291] -> w42
    tunnel: w7 -> [w285]
    tunnel: [w284] -> w14
    stop <- w290 stop-if-true
    # "Init and Dispatcher loop"
    n145 = node-c288() -> (w289:errorcluster)  [unwired: 1 in]
    n146 = Dequeue Element(queue=w294, error in (no error)=w289) -> (queue out=w292:refnum<queue>, element=w293:T17, error out=w288:errorcluster)  [unwired: 1 in, 1 out]
    n147 = case shown="\"Save HW Settings\"" w293 {
      tunnel: [w297 w309 w373 w405 w445 w464 w488 w526 w538 w553 w566 w607 w623 w626 w632 w658 w687 w736] -> w291
      tunnel: w292 -> [w297 w310 w374 w406 w445 w471 w489 w527 w538 w553 w567 w608 w623 w626 w632 w658 w687 w736]
      tunnel: [_ _ _ _ _ _ _ _ _ _ _ _ _ _ _ _ _ TRUE] -> w290
      tunnel: [w296 w306 w380 w435 w446 w465 w486 w525 w539 w552 w564 w602 w622 w625 w628 w657 w684 w727] -> w287
      tunnel: w288 -> [w296 w305 w381 w436 w456 w475 w481 w520 w539 w560 w579 w611 w622 w625 w633 w659 w688 w713]
      tunnel: w285 -> [w295 w298 w355 w409 w460 w461 w476 w515 w535 w542 w563 w601 w621 w624 w634 w660 w681 w726]
      tunnel: [w295 w298 w355 w409 w460 w461 w476 w515 w535 w542 w563 w601 w621 w624 w627 w653 w681 w719] -> w284
      frame Default {
      }
      frame "SW Init" {
        w304 = u8[] [] ("Regions to mark selected")
        w312 = T33 0 items=["no dialog", "OK message", "continue or stop message", "OK message + warnings", "continue/stop + warnings"] ("type of dialog (OK msg:1)")
        n148 = property class="App"(error in=w305) -> (error out=w322:errorcluster, "App.Kind"=w316:T34)  [unwired: 1 in, 1 out]
        n149 = case shown="\"Development System\"" w316 {
          tunnel: [w345 w346 w347] -> w317
          frame "invalid app kind", Default {
            n150 = call <vilib>:"Application Directory.vi"() -> ("Application Directory"=w345:path)
          }
          frame "Run Time System" {
            n151 = call <vilib>:"Application Directory.vi"() -> ("Application Directory"=w346:path)
          }
          frame "Development System" {
            n152 = Current VI's Path() -> (path=w348:path)
            n153 = Strip Path(path=w348) -> (stripped path=w347:path)  [unwired: 1 out]
          }
        }
        n154 = global read "SW_Globals_2.2+.vi" "All references"() -> (w308:T8)
        n155 = Build Path(base path=w317, name or relative path=path "Tracker_settings.tcf") -> (appended path=w332:path)
        n156 = call "SW_Load_settings_to_main_tab_2.vi"("Settings path in"=w332, "Researcher name"="Researcher", "error in (no error)"=w322) -> ("Settings cluster out"=w325:T22, "Settings file path"=w319:path, "error out"=w330:errorcluster)  [unwired: 5 in]
        n157 = global read "SW_Globals_2.2+.vi" "Paths"() -> (w321:T35)
        n158 = global write "SW_Globals_2.2+.vi" "Regions to mark selected"(w304) -> ()
        n159 = call "UI_Set_ByZone_Stim._Control_State_on_Startup.vi"("Error In"=w330, "All references cluster"=w308, "Settings cluster"=w325) -> ("Error Out"=w327:errorcluster, "All references cluster out"=w324:T8, "Regions set for tracking"=w323:u8[], "Settings cluster out"=w326:T22)  [unwired: 4 in, 1 out]
        n160 = Bundle By Name(cluster=w321, "Path to the settings file"=w319) -> (w320:T35)
        n161 = call "SW_Generate_Segmented_Plot_v4_DAQmx.vi"("Settings cluster in"=w326, "Regions to mark set (none)"=w323, "Regions to mark selected (none)"=w304, "Error In"=w327) -> ("Experiment Diagram"=w299:T9, "Settings cluster out"=w329:T22, "Image geometrical and scaling parameters"=w300:T2, "Error Out"=w328:errorcluster)  [unwired: 6 in, 2 out]
        n162 = local write "Img geom and scaling (l.v.o.)"(w300) -> ()
        n163 = local write "Experiment Diagram"(w299) -> ()
        n164 = global write "SW_Globals_2.2+.vi" "Paths"(w320) -> ()
        n165 = call "UI_(01)_Set_startup_controls_state.vi"("error in (no error)"=w328, "Settings cluster in"=w329, "All references in"=w324) -> ("error out"=w314:errorcluster, "Settings cluster out"=w303:T22, "All references out"=w331:T8)
        n166 = Unbundle By Name(w303) -> ("IO parameters"=w301:T25)
        n167 = global write "SW_Globals_2.2+.vi" "All references"(w331) -> ()
        n168 = global write "SW_Globals_2.2+.vi" "Settings cluster"(w303) -> ()
        n169 = call <vilib>:"Simple Error Handler.vi"("error code (no error:0)"=0, "type of dialog (OK msg:1)"=w312, "error in (no error)"=w314) -> ("error?"=w311:bool, "error out"=w307:errorcluster)  [unwired: 2 in, 3 out]
        n170 = call "SW_get_config_of_Zones_and_IO_2.vi"("Sync parameters cluster input"=w301) -> ("Ports IO config (OUT is FALSE)"=w302:bool[])  [unwired: 3 out]
        n171 = case shown="True" w311 {
          tunnel: w310 -> [w337 w344]
          tunnel: [w336 w343] -> w309
          tunnel: w307 -> [w334 w340]
          tunnel: [w333 w341] -> w306
          frame False {
            n172 = Enqueue Element(queue=w337, element=CTL_Control_States."HW Init", error in (no error)=w334) -> (queue out=w336:refnum<queue>, error out=w333:errorcluster)  [unwired: 1 in, 1 out]
          }
          frame True {
            n173 = call <vilib>:"Simple Error Handler.vi"("error in (no error)"=w340) -> ("error out"=w339:errorcluster)  [unwired: 4 in, 4 out]
            n174 = call <vilib>:"Clear Errors.vi"("error in (no error)"=w339) -> ("error out"=w338:errorcluster)  [unwired: 5 in, 1 out]
            n175 = Enqueue Element(queue=w344, element=CTL_Control_States."Close App", error in (no error)=w338) -> (queue out=w343:refnum<queue>, error out=w341:errorcluster)  [unwired: 1 in, 1 out]
          }
        }
        n176 = local write "Ports IO config (l.v.o.)"(w302) -> ()
      }
      frame "HW Init" {
        w369 = T33 0 items=["no dialog", "OK message", "continue or stop message", "OK message + warnings", "continue/stop + warnings"] ("type of dialog (OK msg:1)")
        n177 = call <vilib>:"Set Busy.vi"("error in (no error)"=w381) -> ("error out"=w358:errorcluster)  [unwired: 9 in, 1 out]
        n178 = global read "SW_Globals_2.2+.vi" "All references"() -> (w388:T8)
        n179 = global read "SW_Globals_2.2+.vi" "Settings cluster"() -> (w389:T22)
        n180 = Unbundle By Name(w388) -> ("Indicators references.HW info"=w387:refnum<vi>, "Indicators references.Ready"=w384:refnum<vi>, "Indicators references.Cage size"=w362:refnum<vi>)
        n181 = Unbundle By Name(w389) -> ("Defaults.VISA Resource Name"=w357:string, "Geometry.Cage diameter, mm"=w365:u16)
        n182 = Number To Decimal String(number=w365) -> (decimal integer string=w364:string)  [unwired: 1 in]
        n183 = Concatenate Strings(w364, " mm cage" ("string")) -> (w361:string)
        n184 = property class="Bool (strict)"(reference=w384, error in=w358, "Value"=FALSE, "Colors [4]"=T29 [{"Numeric Control"=16749459, "Numeric Control"=16176658}, {"Numeric Control"=1988894, "Numeric Control"=3381555}, {"Numeric Control"=4934475, "Numeric Control"=7895160}, {"Numeric Control"=994319, "Numeric Control"=1657881}]) -> (reference out=w379:refnum<vi>, error out=w383:errorcluster)
        n185 = property class="Str"(reference=w362, error in=w358, "Value"=w361) -> (error out=w359:errorcluster)  [unwired: 1 out]
        n186 = property on="VISA resource name" class="VISAName"("Value"=w357) -> ()  [unwired: 2 in, 2 out]
        n187 = call "HW_Setup_2.vi"("error in"=w383, "Close port? (F)"=TRUE, "Target FPS"=CTL_Acquisition_speed_selector."Max", "VISA resource name in"=w357) -> ("error out"=w352:errorcluster, "HW information"=w386:string, "Instrument OK?"=w371:bool, "Sync capability"=w378:u8, "SB size"=w356:u8)  [unwired: 3 out]
        n188 = local write "SB size (l.v.o.)"(w356) -> ()
        n189 = Bundle By Name(cluster=w389, "IO parameters.Sync capability"=w378) -> (w385:T22)
        n190 = call <vilib>:"Clear Errors.vi"("error in (no error)"=w352, "specific error code to clear (0: all)"=-1073807346) -> ("error out"=w351:errorcluster, "specific error cleared?"=w349:bool)  [unwired: 4 in]
        n191 = property class="Bool (strict)"(reference=w379, error in=w351, "Value"=w371, "Colors [4]"=T29 [{"Numeric Control"=16749459, "Numeric Control"=16749459}, {"Numeric Control"=1988894, "Numeric Control"=3381555}, {"Numeric Control"=4934475, "Numeric Control"=7895160}, {"Numeric Control"=994319, "Numeric Control"=1657881}]) -> (error out=w375:errorcluster)  [unwired: 1 out]
        n192 = Merge Errors(w375, w359) -> (w360:errorcluster)
        n193 = call <vilib>:"Simple Error Handler.vi"("type of dialog (OK msg:1)"=w369, "error in (no error)"=w360) -> ("error?"=w370:bool, "error out"=w353:errorcluster)  [unwired: 3 in, 3 out]
        n194 = global write "SW_Globals_2.2+.vi" "Settings cluster"(w385) -> ()
        n195 = property on="Property Node" class="Str"(reference=w387, "Value"=w386) -> ()  [unwired: 1 in, 2 out]
        n196 = call <vilib>:"Clear Errors.vi"("error in (no error)"=w353, "specific error code to clear (0: all)"=5002) -> ("error out"=w368:errorcluster)  [unwired: 4 in, 1 out]
        n197 = Or(x=w349, y=w370) -> (x .or. y?=w350:bool)
        n198 = case shown="True" w350 {
          tunnel: [w392 w397] -> w376
          tunnel: w368 -> [w393 w398]
          tunnel: w374 -> [w395 w400]
          tunnel: [w394 w399] -> w373
          frame True {
            n199 = Enqueue Element(queue=w395, element=CTL_Control_States."Re-check HW (init failed)", error in (no error)=w393) -> (queue out=w394:refnum<queue>, error out=w392:errorcluster)  [unwired: 1 in, 1 out]
          }
          frame False {
            n200 = Enqueue Element(queue=w400, element=CTL_Control_States."Update port info (Init OK)", error in (no error)=w398) -> (queue out=w399:refnum<queue>, error out=w397:errorcluster)  [unwired: 1 in, 1 out]
          }
        }
        n201 = call <vilib>:"Unset Busy.vi"("error in (no error)"=w376) -> ("error out"=w380:errorcluster)  [unwired: 10 in]
      }
      frame "Update port info (Init OK)" {
        w431 = 1 items=["Initializing"=-2, "Unknown"=-1, "Not Present"=0, "Present"=1] ("Devices & Chassis:Is Present")
        n202 = call <vilib>:"Set Busy.vi"("error in (no error)"=w436) -> ("error out"=w425:errorcluster)  [unwired: 9 in, 1 out]
        n203 = call <vilib>:"Initialize Session.vi"("error in (no error)"=w425) -> ("error out"=w429:errorcluster, "Session out"=w430:refnum<k21>)  [unwired: 9 in]
        n204 = global read "SW_Globals_2.2+.vi" "All references"() -> (w414:T8)
        n205 = call <vilib>:"Create Filter.vi"("error in (no error)"=w429, "Session in"=w430) -> ("error out"=w433:errorcluster, "Filter out"=w432:refnum<k20>, "Session out"=w428:refnum<k21>)  [unwired: 7 in]
        n206 = global read "SW_Globals_2.2+.vi" "Settings cluster"() -> (w421:T22)
        n207 = property class="System Filter"(reference=w432, error in=w433, "IsPresent"=w431) -> (reference out=w426:refnum<k20>, error out=w427:errorcluster)
        n208 = Unbundle By Name(w414) -> ("Indicators references.Port"=w411:refnum<vi>)
        n209 = Unbundle By Name(w421) -> ("Defaults.VISA Resource Name"=w420:string)
        n210 = call <vilib>:"Find Hardware.vi"("error in (no error)"=w427, "Experts"="ni-visa", "Filter in"=w426, "Session in"=w428) -> ("error out"=w423:errorcluster, "Resources out"=w424:refnum<k20>[], "Session out"=w416:refnum<k21>)  [unwired: 4 in, 1 out]
        n211 = for {
          tunnel: w424 -> [w444] mode=indexing
          tunnel: w423 -> [w443]
          tunnel: [w437] -> w419 mode=indexing if=w440
          tunnel: [w442] -> w422 mode=indexing
          tunnel: w420 -> [w441]
          tunnel: [w439] -> w418 mode=indexing
          n212 = property class="System Hardware"(reference=w444, error in=w443) -> (reference out=w439:refnum<k20>, error out=w442:errorcluster, "PortBinding"=w437:string, "Resource"=w438:string)
          n213 = Equal?(x=w438, y=w441) -> (x = y?=w440:bool)
        }
        n214 = Merge Errors(w422) -> (w417:errorcluster)
        n215 = Index Array(array=w419) -> (element=w413:string)  [unwired: 1 in]
        n216 = Concatenate Strings("port: " ("string"), w413) -> (w410:string)
        n217 = property class="Str"(reference=w411, "Value"=w410) -> ()  [unwired: 1 in, 2 out]
        n218 = call-poly <vilib>:"Close.vi"("error in (no error)"=w417, "Resources in"=w418) -> ("error out"=w415:errorcluster)  [unwired: 9 in]
        n219 = call-poly <vilib>:"Close.vi"("error in (no error)"=w415, "Session in"=w416) -> ("error out"=w408:errorcluster)  [unwired: 9 in]
        n220 = Enqueue Element(queue=w406, element=CTL_Control_States."Save HW Settings", error in (no error)=w408) -> (queue out=w404:refnum<queue>, error out=w403:errorcluster)  [unwired: 1 in, 1 out]
        n221 = Enqueue Element(queue=w404, element=CTL_Control_States."Unlock UI (init OK)", error in (no error)=w403) -> (queue out=w405:refnum<queue>, error out=w402:errorcluster)  [unwired: 1 in, 1 out]
        n222 = call <vilib>:"Unset Busy.vi"("error in (no error)"=w402) -> ("error out"=w435:errorcluster)  [unwired: 10 in]
      }
      frame "Save HW Settings" {
        n223 = global read "SW_Globals_2.2+.vi" "Settings cluster"() -> (w453:T22)
        n224 = global read "SW_Globals_2.2+.vi" "Paths"() -> (w459:T35)
        n225 = Unbundle By Name(w453) -> ("Defaults"=w452:T36)
        n226 = Unbundle By Name(w459) -> ("Path to the settings file"=w458:path)
        n227 = Flatten To XML(anything=w452) -> (xml string=w451:string)
        n228 = call <vilib>:"Open Config Data.vi"("error in (no error)"=w456, "create file if necessary (T)"=FALSE, "configuration file path"=w458) -> ("error out"=w450:errorcluster, "refnum"=w455:T37)  [unwired: 6 in, 1 out]
        n229 = call "SW_Save_parameter_group.vi"("Settings file refnum in"=w455, "error in"=w450, "Parameter value"=w451, "Param group"="Defaults", "Researcher name"="Researcher") -> ("error out"=w448:errorcluster, "Settings file refnum out"=w447:T37)  [unwired: 4 in, 1 out]
        n230 = call <vilib>:"Close Config Data.vi"("error in (no error)"=w448, "refnum"=w447) -> ("error out"=w446:errorcluster)  [unwired: 8 in, 1 out]
      }
      frame "Unlock UI (init OK)" {
        n231 = global read "SW_Globals_2.2+.vi" "Settings cluster"() -> (w473:T22)
        n232 = global read "SW_Globals_2.2+.vi" "All references"() -> (w474:T8)
        n233 = call "UI_(02)_Unlock.vi"("error in (no error)"=w475, "Settings cluster in"=w473, "All references in"=w474) -> ("error out"=w472:errorcluster)  [unwired: 2 out]
        n234 = Enqueue Element(queue=w471, element=CTL_Control_States."Zones layout update", error in (no error)=w472) -> (queue out=w468:refnum<queue>, error out=w469:errorcluster)  [unwired: 1 in, 1 out]
        n235 = Enqueue Element(queue=w468, element=CTL_Control_States."Upd. trace length", error in (no error)=w469) -> (queue out=w463:refnum<queue>, error out=w466:errorcluster)  [unwired: 1 in, 1 out]
        n236 = Enqueue Element(queue=w463, element=CTL_Control_States."Update filter", error in (no error)=w466) -> (queue out=w464:refnum<queue>, error out=w465:errorcluster)  [unwired: 1 in, 1 out]
      }
      frame "Re-check HW (init failed)" {
        w484 = enum32{"Settings", "Recording and Analysis"}."Settings" ("Value")
        n237 = global read "SW_Globals_2.2+.vi" "All references"() -> (w499:T8)
        n238 = Unbundle By Name(w499) -> ("Controls references.Set, Rec and Analyse Tab"=w485:refnum<vi>, "Indicators references.Ready"=w496:refnum<vi>, "Controls references.Check HW connection"=w495:refnum<vi>)
        n239 = property class="TabCtl (strict)"(reference=w485, error in=w481, "Value"=w484) -> (error out=w478:errorcluster, "Pages"=w482:refnum<vi>[])  [unwired: 1 out]
        n240 = To Long Integer(number=w484) -> (32bit integer=w483:i32)
        n241 = Index Array(array=w482, index=w483) -> (element=w480:refnum<vi>)
        n242 = property class="Page"(reference=w480, error in=w478, "PageEnb"=T31."Page Enabled" ("Page Enabled State")) -> (error out=w477:errorcluster)  [unwired: 1 out]
        n243 = property class="Bool"(reference=w495, error in=w477, "DisabledEnum"=T32."Enabled" ("Disabled")) -> (error out=w493:errorcluster)  [unwired: 1 out]
        n244 = property class="Bool (strict)"(reference=w496, error in=w493, "Value"=FALSE, "Colors [4]"=T29 [{"Numeric Control"=16749459, "Numeric Control"=16749459}, {"Numeric Control"=1988894, "Numeric Control"=3381555}, {"Numeric Control"=4934475, "Numeric Control"=7895160}, {"Numeric Control"=994319, "Numeric Control"=1657881}]) -> (error out=w492:errorcluster)  [unwired: 1 out]
        n245 = call "Display Message to User"("error in (no error)"=w492, "Enable"=TRUE) -> ("error out"=w487:errorcluster, "Retry"=w490:bool)  [unwired: 8 in]
        n246 = case shown="True" w490 {
          tunnel: w489 -> [w504 w509]
          tunnel: [w503 w508] -> w488
          tunnel: w487 -> [w502 w507]
          tunnel: [w501 w506] -> w486
          frame True {
            # "Re-check automatically"
            n247 = Enqueue Element(queue=w504, element=CTL_Control_States."HW Init", error in (no error)=w502) -> (queue out=w503:refnum<queue>, error out=w501:errorcluster)  [unwired: 1 in, 1 out]
          }
          frame False {
            # "Pop-up manual port adjustment dialog"
            n248 = Enqueue Element(queue=w509, element=CTL_Control_States."Configure port(s)", error in (no error)=w507) -> (queue out=w508:refnum<queue>, error out=w506:errorcluster)  [unwired: 1 in, 1 out]
          }
        }
      }
      frame "Configure port(s)" {
        w523 = enum32{"Settings", "Recording and Analysis"}."Settings" ("Value")
        # "Module not finished yet"
        n249 = global read "SW_Globals_2.2+.vi" "All references"() -> (w534:T8)
        n250 = Unbundle By Name(w534) -> ("Controls references.Set, Rec and Analyse Tab"=w524:refnum<vi>, "Indicators references.Ready"=w531:refnum<vi>, "Controls references.Check HW connection"=w530:refnum<vi>)
        n251 = property class="TabCtl (strict)"(reference=w524, error in=w520, "Value"=w523) -> (error out=w517:errorcluster, "Pages"=w521:refnum<vi>[])  [unwired: 1 out]
        n252 = To Long Integer(number=w523) -> (32bit integer=w522:i32)
        n253 = Index Array(array=w521, index=w522) -> (element=w519:refnum<vi>)
        n254 = property class="Page"(reference=w519, error in=w517, "PageEnb"=T31."Page Enabled" ("Page Enabled State")) -> (error out=w516:errorcluster)  [unwired: 1 out]
        n255 = property class="Bool"(reference=w530, error in=w516, "DisabledEnum"=T32."Enabled" ("Disabled")) -> (error out=w528:errorcluster)  [unwired: 1 out]
        n256 = global read "SW_Globals_2.2+.vi" "Settings cluster"() -> (w512:T22)
        n257 = property class="Bool (strict)"(reference=w531, error in=w528, "Value"=FALSE, "Colors [4]"=T29 [{"Numeric Control"=16749459, "Numeric Control"=16749459}, {"Numeric Control"=1988894, "Numeric Control"=3381555}, {"Numeric Control"=4934475, "Numeric Control"=7895160}, {"Numeric Control"=994319, "Numeric Control"=1657881}]) -> (error out=w514:errorcluster)  [unwired: 1 out]
        n258 = call "HW_Configure_port(s).vi"("Settings cluster in"=w512, "error in (no error)"=w514) -> ("Settings cluster out"=w511:T22, "error out"=w513:errorcluster)  [unwired: 1 out]
        n259 = global write "SW_Globals_2.2+.vi" "Settings cluster"(w511) -> ()
        n260 = Enqueue Element(queue=w527, element=CTL_Control_States."HW Init", error in (no error)=w513) -> (queue out=w526:refnum<queue>, error out=w525:errorcluster)  [unwired: 1 in, 1 out]
      }
      frame "Update filter" {
        n261 = global read "SW_Globals_2.2+.vi" "Settings cluster"() -> (w537:T22)
        n262 = Unbundle By Name(w537) -> ("Recording and saving.Data filtering"=w536:T23)
        n263 = call "SW_SG_coefficients.vi"("1st order derivative? (F)"=FALSE, "Filter parameters"=w536) -> ("SG filter coefficients"=w540:dbl[])  [unwired: 1 in]
        n264 = local write "SG coeff. 0th order (l.v.o.)"(w540) -> ()
      }
      frame "Zones layout update" {
        n265 = global read "SW_Globals_2.2+.vi" "All references"() -> (w556:T8)
        n266 = Unbundle By Name(w556) -> ("Controls references.Show zones"=w555:refnum<vi>, "Controls references.Show magnets"=w554:refnum<vi>)
        n267 = global read "SW_Globals_2.2+.vi" "Settings cluster"() -> (w561:T22)
        n268 = global read "SW_Globals_2.2+.vi" "Regions to mark selected"() -> (w547:u8[])
        n269 = property class="Bool (strict)"(reference=w555) -> ("Value"=w543:bool)  [unwired: 1 in, 2 out]
        n270 = Select(t=T32."Disabled and Grayed Out" ("Disabled"), s=w543, f=T32."Enabled" ("Disabled")) -> (s? t:f=w548:T32)
        n271 = property class="Bool (strict)"(reference=w554, "DisabledEnum"=w548) -> ("Value"=w551:bool)  [unwired: 1 in, 2 out]
        n272 = call "UI_Set_ByZone_Stim._Control_State_on_Startup.vi"("Error In"=w560, "Regions to mark selected in"=w547, "All references cluster"=w556, "Settings cluster"=w561) -> ("Error Out"=w557:errorcluster, "Regions to mark selected out"=w546:u8[], "Regions set for tracking"=w559:u8[], "Settings cluster out"=w558:T22)  [unwired: 3 in, 1 out]
        n273 = call "SW_Generate_Segmented_Plot_v4_DAQmx.vi"("Settings cluster in"=w558, "Regions to mark set (none)"=w559, "Regions to mark selected (none)"=w546, "Error In"=w557, "Show magnets (T)"=w551, "Show zones (T)"=w543) -> ("Experiment Diagram"=w562:T9, "Image geometrical and scaling parameters"=w545:T2, "Error Out"=w552:errorcluster)  [unwired: 4 in, 3 out]
        n274 = Not(x=w543) -> (.not. x?=w544:bool)
        n275 = global write "SW_Globals_2.2+.vi" "Regions to mark selected"(w546) -> ()
        n276 = local write "Bright mouse lineout (l.v.o.)"(w544) -> ()
        n277 = property on="Experiment Diagram" class="ImageControl"("Value"=w562) -> ()  [unwired: 2 in, 2 out]
        n278 = local write "Img geom and scaling (l.v.o.)"(w545) -> ()
      }
      frame "Set I/O config" {
        n279 = global read "SW_Globals_2.2+.vi" "Settings cluster"() -> (w571:T22)
        n280 = global read "SW_Globals_2.2+.vi" "All references"() -> (w582:T8)
        n281 = Unbundle By Name(w571) -> ("Defaults.VISA Resource Name"=w578:string, "IO parameters"=w583:T25, "IO parameters.Sync capability"=w573:u8)
        n282 = Unbundle By Name(w582) -> ("Indicators references.IO status indicator"=w581:refnum<vi>)
        n283 = call "HW_set_IO_ports_3-pos_2.vi"("IO parameters cluster"=w583) -> ("IO parameters cluster output"=w570:T25, "IO changed"=w568:bool)
        n284 = call "SW_get_IO_ports_representation_2.vi"("Sync parameters cluster input"=w570) -> ("IO status indicator"=w580:T12)
        n285 = call "SW_get_config_of_Zones_and_IO_2.vi"("Sync parameters cluster input"=w570) -> ("Ports IO config (OUT is FALSE)"=w577:bool[], "IO inversion config."=w576:u16)  [unwired: 2 out]
        n286 = property class="Clust"(reference=w581, error in=w579, "Value"=w580) -> (error out=w575:errorcluster)  [unwired: 1 out]
        n287 = Bundle By Name(cluster=w571, "IO parameters"=w570) -> (w569:T22)
        n288 = call "HW_Set_IO_Dir_on_ECU.vi"("Error In"=w575, "IO ports config"=w577, "VISA resource name"=w578, "IO inversion config."=w576) -> ("error out"=w572:errorcluster, "VISA resource name out"=w574:refnum<visa-resource-name>)
        n289 = case shown="1.." w573 {
          tunnel: w574 -> [_ w600]
          tunnel: w572 -> [w591 w599]
          tunnel: w570 -> [_ w598]
          tunnel: [w591 w592] -> w565
          frame 0, Default {
          }
          frame 1.. {
            w595 = u16 4
            n290 = Unbundle By Name(w598) -> ("IO 1 configuration"=w597:u16, "IO 2 configuration"=w596:u16)
            n291 = Equal?(x=w597, y=w595) -> (x = y?=w594:bool)
            n292 = Equal?(x=w596, y=w595) -> (x = y?=w593:bool)
            n293 = call "HW_Set_SYNC_Status.vi"("error in (no error)"=w599, "SYNC 2"=w593, "SYNC 1"=w594, "VISA Resource name IN"=w600) -> ("error out"=w592:errorcluster)  [unwired: 6 in, 1 out]
          }
        }
        n294 = global write "SW_Globals_2.2+.vi" "Settings cluster"(w569) -> ()
        n295 = case shown="True" w568 {
          tunnel: w567 -> [w585 w586]
          tunnel: [w585 w588] -> w566
          tunnel: w565 -> [w584 w590]
          tunnel: [w584 w587] -> w564
          frame False {
            # "IO not changed"
          }
          frame True {
            # "IO changed"
            n296 = Enqueue Element(queue=w586, element=CTL_Control_States."Reset stimulus", error in (no error)=w590) -> (queue out=w588:refnum<queue>, error out=w587:errorcluster)  [unwired: 1 in, 1 out]
          }
        }
      }
      frame "Cage and recording settings" {
        n297 = call "SW_Set_Cage_and_Recording_Settings.vi"("error in (no error)"=w611) -> ("error out"=w610:errorcluster)  [unwired: 2 in]
        n298 = Enqueue Element(queue=w608, element=CTL_Control_States."Zones layout update", error in (no error)=w610) -> (queue out=w606:refnum<queue>, error out=w609:errorcluster)  [unwired: 1 in, 1 out]
        n299 = Enqueue Element(queue=w606, element=CTL_Control_States."Update filter", error in (no error)=w609) -> (queue out=w607:refnum<queue>, error out=w603:errorcluster)  [unwired: 1 in, 1 out]
        n300 = flat-sequence {
          tunnel: w603 -> [w613]
          tunnel: [w612] -> w602
          frame #0 {
            n301 = global read "SW_Globals_2.2+.vi" "Settings cluster"() -> (w618:T22)
            n302 = global read "SW_Globals_2.2+.vi" "All references"() -> (w616:T8)
            n303 = Unbundle By Name(w616) -> ("Indicators references.Cage size"=w615:refnum<vi>)
            n304 = Unbundle By Name(w618) -> ("Geometry.Cage diameter, mm"=w617:u16)
            n305 = Number To Decimal String(number=w617) -> (decimal integer string=w620:string)  [unwired: 1 in]
            n306 = Concatenate Strings(w620, " mm cage" ("string")) -> (w614:string)
            n307 = property class="Str"(reference=w615, error in=w613, "Value"=w614) -> (error out=w612:errorcluster)  [unwired: 1 out]
          }
        }
      }
      frame "Reset stimulus" {
      }
      frame "Reset zones" {
      }
      frame "Play Start" {
        n308 = Get Notifier Status(notifier=w634, error in (no error)=w633) -> (notifier out=w631:refnum<notifier>, current notification=w630:T16, error out=w635:errorcluster)  [unwired: 2 out]
        n309 = Unbundle By Name(w630) -> ("Data loaded"=w629:bool)
        n310 = case shown="False" w629 {
          tunnel: w635 -> [w645 w652]
          tunnel: [w639 w652] -> w628
          tunnel: w631 -> [w649 w651]
          tunnel: w630 -> [w648 _]
          tunnel: [w636 w651] -> w627
          frame False {
            # "This part is running when working online"
            n311 = global read "SW_Globals_2.2+.vi" "Settings cluster"() -> (w638:T22)
            n312 = Unbundle By Name(w638) -> ("Defaults.VISA Resource Name"=w646:string)
            n313 = call "HW_Acquisition_Start.vi"("Error In"=w645, "VISA resource name in"=w646) -> ("Error Out"=w642:errorcluster)  [unwired: 1 out]
            n314 = global read "SW_Globals_2.2+.vi" "All references"() -> (w637:T8)
            n315 = Unbundle By Name(w637) -> ("Controls references.Play/Pause"=w644:refnum<vi>)
            n316 = property class="Bool (strict)"(reference=w644, error in=w642, "Value"=TRUE) -> (error out=w641:errorcluster)  [unwired: 1 out]
            n317 = Bundle By Name(cluster=w648, "Acq. is ON"=TRUE ("\"Play\" is ON")) -> (w647:T16)
            n318 = Send Notification(notification=w647, notifier=w649, error in (no error)=w641) -> (notifier out=w636:refnum<notifier>, error out=w640:errorcluster)
            n319 = call "UI_(03A)_Set_Play_State.vi"("error in (no error)"=w640, "Settings cluster in"=w638, "All references in"=w637) -> ("error out"=w639:errorcluster)  [unwired: 2 out]
          }
          frame True {
            # "This part is running when working with the recorded data"
          }
        }
      }
      frame "Play Stop" {
        n320 = Get Notifier Status(notifier=w660, error in (no error)=w659) -> (notifier out=w656:refnum<notifier>, current notification=w655:T16, error out=w661:errorcluster)  [unwired: 2 out]
        n321 = Unbundle By Name(w655) -> ("Data loaded"=w654:bool)
        n322 = case shown="True" w654 {
          tunnel: w661 -> [w671 w678]
          tunnel: [w665 w678] -> w657
          tunnel: w656 -> [w675 w677]
          tunnel: w655 -> [w674 _]
          tunnel: [w662 w677] -> w653
          frame False {
            # "This part is running when working online"
            n323 = Bundle By Name(cluster=w674, "Acq. is ON"=FALSE ("\"Play\" is ON")) -> (w673:T16)
            n324 = global read "SW_Globals_2.2+.vi" "Settings cluster"() -> (w664:T22)
            n325 = Send Notification(notification=w673, notifier=w675, error in (no error)=w671) -> (notifier out=w662:refnum<notifier>, error out=w670:errorcluster)
            n326 = Unbundle By Name(w664) -> ("Defaults.VISA Resource Name"=w672:string)
            n327 = call "HW_Acquisition_Stop.vi"("Error In"=w670, "VISA resource name in"=w672) -> ("Error Out"=w667:errorcluster)  [unwired: 1 out]
            n328 = global read "SW_Globals_2.2+.vi" "All references"() -> (w663:T8)
            n329 = Unbundle By Name(w663) -> ("Controls references.Play/Pause"=w669:refnum<vi>)
            n330 = property class="Bool (strict)"(reference=w669, error in=w667, "Value"=FALSE) -> (error out=w666:errorcluster)  [unwired: 1 out]
            n331 = call "UI_(04A)_Set_Stop_State.vi"("error in (no error)"=w666, "Settings cluster in"=w664, "All references in"=w663) -> ("error out"=w665:errorcluster)  [unwired: 2 out]
          }
          frame True {
            # "This part is running when working with the recorded data"
          }
        }
      }
      frame "Upd. trace length" {
        w691 = u32[] [255, 65535, 6618880, 16776960, 16744448, 16711680] ("Initial colors ramp array")
        n332 = global read "SW_Globals_2.2+.vi" "All references"() -> (w704:T8)
        n333 = local read "UI update period (l.v.o.)"() -> (w702:i64)
        n334 = Unbundle By Name(w704) -> ("Controls references.Trace, s"=w703:refnum<vi>, "Controls references.Rainbow track"=w686:refnum<vi>)
        n335 = To Double Precision Float(number=i64 1000 ("x")) -> (double precision float=w680:dbl)
        n336 = Array Size(array=w691) -> (size(s)=w692:i32)
        n337 = To Double Precision Float(number=w702) -> (double precision float=w679:dbl)
        n338 = Decrement(x=w692) -> (x-1=w696:i32)
        n339 = Divide(x=w680, y=w679) -> (x/y=w699:dbl)
        n340 = property class="Slide (strict)"(reference=w703, error in=w688) -> (error out=w685:errorcluster, "Value"=w700:u16)  [unwired: 1 out]
        n341 = Multiply(x=w700, y=w699) -> (x*y=w698:dbl)
        n342 = To Unsigned Word Integer(number=w698) -> (unsigned 16bit integer=w690:u16)
        n343 = Decrement(x=w690) -> (x-1=w693:u16)
        n344 = Divide(x=w693, y=w696) -> (x/y=w697:dbl)
        n345 = for {
          N: w692 -> [_]
          tunnel: [w707] -> w695 mode=indexing
          tunnel: w693 -> [w711]
          tunnel: w697 -> [w709]
          workers-P: _ -> [_]
          i -> [w708]
          n346 = To Double Precision Float(number=w708) -> (double precision float=w705:dbl)
          n347 = To Double Precision Float(number=w711) -> (double precision float=w706:dbl)
          n348 = Multiply(x=w709, y=w705) -> (x*y=w710:dbl)
          n349 = Subtract(x=w706, y=w710) -> (x-y=w707:dbl)
        }
        n350 = Reverse 1D Array(array=w695) -> (reversed array=w694:dbl[])
        n351 = local write "Trace length, samples (l.v.o)"(w690) -> ()
        n352 = property class="Bool (strict)"(reference=w686, error in=w685) -> (error out=w683:errorcluster, "Value"=w682:bool)  [unwired: 1 out]
        n353 = call "SW_Generate_Color_Ramp.vi"("Colors rel. pos."=w694, "Colors array"=w691) -> ("Colors array"=w689:u32[])
        n354 = local write "Colors array (l.v.o.)"(w689) -> ()
        n355 = local write "Rainbow track (l.v.o.)"(w682) -> ()
        n356 = Merge Errors(w685, w683) -> (w684:errorcluster)
      }
      frame "Close App" {
        w730 = T38 128 items=["Flush Receive Buffer"=16, "Write Transmit Buffer to Device"=32, "Flush Receive Buffer (No I/O)"=64, "Flush Transmit Buffer"=128] ("Mask")
        n357 = global read "SW_Globals_2.2+.vi" "Settings cluster"() -> (w729:T22)
        n358 = Unbundle By Name(w729) -> ("Defaults.VISA Resource Name"=w715:string)
        n359 = call "HW_Acquisition_Stop.vi"("Error In"=w713, "VISA resource name in"=w715) -> ("Error Out"=w712:errorcluster, "VISA resource name out"=w714:refnum<visa-resource-name>)
        n360 = VISA Flush I/O Buffer(VISA resource name=w714, mask (16)=w730, error in (no error)=w712) -> (VISA resource name out=w731:refnum<visa-resource-name>, error out=w732:errorcluster)
        n361 = VISA Clear(VISA resource name=w731, error in (no error)=w732) -> (VISA resource name out=w734:refnum<visa-resource-name>, error out=w733:errorcluster)
        n362 = VISA Close(VISA resource name=w734, error in (no error)=w733) -> (error out=w735:errorcluster)
        n363 = call <vilib>:"Clear Errors.vi"("error in (no error)"=w735) -> ("error out"=w725:errorcluster)  [unwired: 5 in, 1 out]
        n364 = Get Notifier Status(notifier=w726, error in (no error)=w725) -> (notifier out=w723:refnum<notifier>, current notification=w722:T16, error out=w724:errorcluster)  [unwired: 2 out]
        n365 = Bundle By Name(cluster=w722, "Stop and Exit"=TRUE) -> (w721:T16)
        n366 = Send Notification(notification=w721, notifier=w723, error in (no error)=w724) -> (notifier out=w719:refnum<notifier>, error out=w718:errorcluster)
        n367 = flat-sequence {
          tunnel: w718 -> [w742]
          tunnel: [w742] -> w717
          frame #0 {
            n368 = Wait (ms)(milliseconds to wait=u32 250) -> ()  [unwired: 1 out]
          }
        }
        n369 = property class="App"() -> ("App.Kind"=w716:T34)  [unwired: 2 in, 2 out]
        n370 = case shown="\"Development System\"" w716 {
          tunnel: [w738 w741] -> w727
          tunnel: w717 -> [w737 w741]
          frame "invalid app kind", Default {
            # "Close FP only if app is compiled"
            n371 = global read "SW_Globals_2.2+.vi" "All references"() -> (w740:T8)
            n372 = Unbundle By Name(w740) -> ("Service references.This VI"=w739:refnum<vi>)
            n373 = invoke class="VI" method="FP.Close"(reference=w739, error in=w737) -> (error out=w738:errorcluster)  [unwired: 1 in, 2 out]
          }
          frame "Development System" {
          }
        }
      }
    }
    n374 = call <vilib>:"Simple Error Handler.vi"("error in (no error)"=w287) -> ("error out"=w286:errorcluster)  [unwired: 4 in, 4 out]
    n375 = node-c288(w286) -> ()  [unwired: 1 out]
  }
  n376 = timed-loop {
    timing: w35 -> [_]
    timing-out: [_] -> w34
    tunnel: w6 -> [_]
    tunnel: w7 -> [w759]
    border: "" -> [_]
    tunnel: [w751] -> w24
    stop <- w757 stop-if-true
    # "Data gathering and initial processing loop"
    n377 = node-c288() -> (w749:errorcluster)  [unwired: 1 in]
    n378 = Get Notifier Status(notifier=w759, error in (no error)=w749) -> (current notification=w758:T16, error out=w750:errorcluster)  [unwired: 3 out]
    n379 = Unbundle By Name(w758) -> ("Acq. is ON"=w755:bool, "Stop and Exit"=w757:bool)
    n380 = case shown="True" w755 {
      tunnel: w750 -> [w760 w768]
      tunnel: [w760 w762] -> w752
      tunnel: [_ w761] -> w751
      frame False {
      }
      frame True {
        n381 = local read "VISA resource name"() -> (w766:refnum<visa-resource-name>)
        n382 = call "HW_Get_data_flow_from_serial_port.vi"("error in"=w768, "VISA resource name in"=w766) -> ("Not empty?"=w767:bool, "error out"=w763:errorcluster, "Timestamp"=w764:timestamp, "Data"=w765:string)  [unwired: 2 in, 1 out]
        n383 = case shown="True" w767 {
          tunnel: w765 -> [_ w781]
          tunnel: w764 -> [_ w780]
          tunnel: w763 -> [w769 w784]
          tunnel: [w769 w775] -> w762
          tunnel: [_ w770] -> w761
          frame False {
          }
          frame True {
            n384 = global read "SW_Globals_2.2+.vi" "Settings cluster"() -> (w772:T22)
            n385 = local read "Ports IO config (l.v.o.)"() -> (w778:bool[])
            n386 = local read "SB size (l.v.o.)"() -> (w771:u8)
            n387 = feedback #1() -> (w782:string)
            n388 = Concatenate Strings(w782, w781) -> (w779:string)
            n389 = Unbundle By Name(w772) -> ("IO parameters.IO inversion config."=w777:u16)
            n390 = call "FL_Decode_RAW_to_DEC_2.vi"("SB size (loc. var. only)"=w771, "IO ports config"=w778, "Input string"=w779, "Input timestamp"=w780, "IO inversion config."=w777, "Error In"=w784) -> ("Output string leftover"=w783:string, "DEC output cluster"=w774:T39, "Error Out"=w776:errorcluster)
            n391 = feedback-in #1(w783) -> ()
            n392 = Unbundle By Name(w774) -> ("Frame OK"=w773:bool)
            n393 = case shown="True" w773 {
              tunnel: w774 -> [_ w800]
              tunnel: w776 -> [w785 w789]
              tunnel: [w785 w789] -> w775
              tunnel: w772 -> [_ w797]
              tunnel: w771 -> [_ w792]
              tunnel: [_ w787] -> w770
              frame False {
              }
              frame True {
                n394 = local read "SG coeff. 0th order (l.v.o.)"() -> (w795:dbl[])
                n395 = Unbundle By Name(w797) -> ("Geometry.Bridge H. offset"=w799:sgl, "Geometry.Bridge V. offset"=w798:sgl, "Geometry.Alt. magn. orientation"=w786:bool, "Geometry.Twisted neck"=w790:bool, "Geometry.Bridge swap"=w791:bool)
                n396 = call "FL_Adjust_raw_magnets_coords.vi"("Offset H."=w799, "Offset V."=w798, "Alternative magnets orientation"=w786, "DEC cluster in"=w800) -> ("DEC cluster out"=w796:T40)  [unwired: 3 in]
                n397 = call "FL_DEC_split_2_and_prefilter.vi"("DEC input cluster"=w796, "SG filter coefficients"=w795) -> ("Magnets coords"=w794:cluster{"X1":dbl, "Y1":dbl, "X2":dbl, "Y2":dbl})  [unwired: 1 in, 3 out]
                n398 = call "FL_Calculate_Coordinates_Diff_R_Center.vi"("Magnets coords in"=w794) -> ("Output cluster of data"=w793:T41)  [unwired: 2 in]
                n399 = call "FL_Calculate_phi_theta_etc_2.vi"("Input cluster of data"=w793, "SB size"=w792, "Bridge swap"=w791, "Use alternative magnets orientation"=w786, "Twisted neck"=w790) -> ("Animal coordinates"=w788:T42)  [unwired: 1 in]
                n400 = call <extravilib>:"Write.vi"("element"=w788) -> ("channel"=w787:T43)  [unwired: 8 in, 2 out]
              }
            }
          }
        }
      }
    }
    n401 = Select(t=i64 1, s=w755, f=i64 101) -> (s? t:f=w754:i64)
    n402 = node-c288(w752, w754) -> ()  [unwired: 1 out]
  }
  n403 = timed-loop {
    timing: w28 -> [_]
    timing-out: [_] -> w27
    tunnel: w6 -> [_]
    tunnel: w7 -> [w820]
    tunnel: w24 -> [w819]
    stop <- w814 stop-if-true
    # "UI drawings and plots update loop"
    n404 = node-c288() -> (w817:errorcluster)  [unwired: 1 in]
    n405 = call <extravilib>:"Read.vi"("channel"=w819, "timeout in ms (-1)"=563) -> ("element"=w818:T42, "count"=w808:i32, "timed out?"=w813:bool)  [unwired: 4 in, 3 out]
    n406 = Get Notifier Status(notifier=w820, error in (no error)=w817) -> (current notification=w821:T16, error out=w816:errorcluster)  [unwired: 3 out]
    n407 = Unbundle By Name(w821) -> ("Stop and Exit"=w814:bool)
    n408 = Not(x=w813) -> (.not. x?=w810:bool)
    n409 = Equal To 0?(x=w808) -> (x = 0?=w811:bool)
    n410 = Not(x=w814) -> (.not. x?=w812:bool)
    n411 = Compound Arithmetic op=AND(w810, w811, w812) -> (w809:bool)
    n412 = case shown="True" w809 {
      tunnel: w818 -> [_ w828]
      frame False {
      }
      frame True {
        n413 = local read "Bright mouse lineout (l.v.o.)"() -> (w823:bool)
        n414 = local read "Experiment Diagram"() -> (w827:T9)
        n415 = local read "Rainbow track (l.v.o.)"() -> (w822:bool)
        n416 = local read "Trace length, samples (l.v.o)"() -> (w825:u16)
        n417 = local read "Img geom and scaling (l.v.o.)"() -> (w830:T2)
        n418 = local read "Colors array (l.v.o.)"() -> (w824:u32[])
        n419 = Unbundle By Name(w830) -> ("Pixels per mm"=w829:dbl)
        n420 = call "SW_Draw_mouse_DAQmx.vi"("Image In"=w827, "Pixels per mm"=w829, "Mouse position"=w828, "Trace length, samples"=w825, "Bright mouse lineout"=w823, "Colors array input"=w824, "Rainbow colors"=w822) -> ("Image Out"=w826:T9)  [unwired: 8 in]
        n421 = local write "Experiment Diagram"(w826) -> ()
      }
    }
    n422 = local read "UI update period (l.v.o.)"() -> (w807:i64)
    n423 = node-c288(w816, w807) -> ()  [unwired: 1 out]
  }
  n424 = timed-loop {
    timing: w13 -> [_]
    timing-out: [_] -> w12
    tunnel: w7 -> [w851]
    tunnel: w6 -> [w840]
    tunnel: w1 -> [w845]
    stop <- w848 stop-if-true
    # "Whatchdog loop"
    n425 = node-c288() -> (w850:errorcluster, w846:i64)  [unwired: 1 in]
    n426 = Get Notifier Status(notifier=w851, error in (no error)=w850) -> (current notification=w849:T16, error out=w847:errorcluster)  [unwired: 3 out]
    n427 = local read "UI update period (l.v.o.)"() -> (w843:i64)
    n428 = call "SW_Get_CPU_load.vi"("error in (no error)"=w847, "Buffer length, sec"=5.0, "Scan interval, ms"=w846, "CPU monitor .NET reference in"=w845) -> ("error out"=w839:errorcluster, "Historical CPU load, %"=w837:sgl)  [unwired: 2 out]
    n429 = call "SW_Adjust_UI_draw_interwal.vi"("UI update period (l.v.o.) in"=w843, "Historical CPU load, %"=w837) -> ("Updated?"=w841:bool, "UI update period (l.v.o.) out"=w842:i64)
    n430 = Unbundle By Name(w849) -> ("Stop and Exit"=w848:bool)
    n431 = local write "CPU load"(w837) -> ()
    n432 = local write "UI update period (l.v.o.)"(w842) -> ()
    n433 = case shown="True" w841 {
      tunnel: w840 -> [_ w855]
      tunnel: w839 -> [w852 w854]
      tunnel: [w852 w853] -> w838
      frame False {
        # "No update"
      }
      frame True {
        # "Update trace length"
        n434 = Enqueue Element(queue=w855, element=CTL_Control_States."Upd. trace length", error in (no error)=w854) -> (error out=w853:errorcluster)  [unwired: 1 in, 2 out]
      }
    }
    n435 = node-c288(w838) -> ()  [unwired: 1 out]
  }
  n436 = node-c288(w12) -> (w4:errorcluster)
  n437 = node-c288(w27) -> (w18:errorcluster)
  n438 = node-c288(w39) -> (w19:errorcluster)
  n439 = node-c288(w34) -> (w20:errorcluster)
  n440 = Merge Errors(w18, w4) -> (w5:errorcluster)
  n441 = node-c288(w46) -> (w21:errorcluster)
  n442 = Flush Queue(queue=w42, error in (no error)=w21) -> (queue out=w41:refnum<queue>, error out=w22:errorcluster)  [unwired: 1 out]
  n443 = Release Queue(queue=w41, error in (no error)=w22) -> (error out=w17:errorcluster)  [unwired: 1 in, 2 out]
  n444 = Merge Errors(w17, w19, w20, w5) -> (w16:errorcluster)
  n445 = Release Notifier(notifier=w14, error in (no error)=w16) -> (error out=→"error out":errorcluster)  [unwired: 1 in, 2 out]
